vi "main.vi"() -> ()   [LabVIEW 2018]
uses:
  SubVIs_Dental robot/Type Define/Commmands.ctl
  SubVIs_Dental robot/Type Define/Main Pages.ctl
  <vilib>/Platform/TimedLoop/XDataNode/timing_clust.ctl
  <vilib>/Platform/TimedLoop/XDataNode/nitl_modes.ctl
  <vilib>/Platform/TimedLoop/XDataNode/wakeup.ctl
  <vilib>/Analysis/_algsub.llb/Vector Norm Type.ctl
  <vilib>/Analysis/baseanly.llb/A x Vector.vi
  a7223f14-2dee-44f5-bb18-0364424e4be1.vi
  0510b20e-cdd4-4c00-a2e4-b6458116f7e6.vi
  6765c77a-608f-47a9-82f1-7d78e4eb0e2c.vi
  9b5042e6-a8af-4737-a7d5-6a0044b5b849.vi
  4ad8b042-512e-4ff8-852c-0cd1c3cad4b9.vi
  86f0d0e6-1215-4d7f-931e-98a8c43bff1f.vi
  f29c3c44-4b71-459f-8cb8-0042c545ba9a.vi
  d7c4ca3e-ecce-44e0-a421-952e676fecf6.vi
  981894b4-ccec-4f9d-89cc-fdaa1394f8a6.vi
  9c9e3e7b-044e-4f20-b28a-2f2dc11135a4.vi
  9fd7527a-2d21-4efb-8458-bb367c16f289.vi
  ac7faa24-f845-40ca-90b7-81be7ed5a357.vi
  b63aa834-2712-49f4-8037-f59c6ffc9581.vi
  f501b187-2088-4d7b-8b35-1f4e4e40070a.vi
  <vilib>/Analysis/_algsub.llb/Real Vector Norm.vi
  bbe701d4-6856-4238-8169-f1a63681c652.vi
  2e5cd8ad-a022-48e3-a566-60a3cbf6d178.vi
  11c04ccb-2e07-4f2a-b784-9dc4474bd3c3.vi
  df89aa8a-d510-48a8-89d6-09f8ad9d1347.vi
  c9b8846e-2642-4342-81ce-7650c1843fd3.vi
  e93a78a8-cf73-409a-8246-49de62ed042d.vi
  3db6b772-aa7e-4faf-b327-bcfc711d862c.vi
  947c7df0-b853-4919-9a27-33aee5587755.vi
  376b9600-9bf4-49ac-95b6-11595f89b64b.vi
  2f109b7a-7238-4649-a91e-82c40714c455.vi
  015dea3f-de33-43d8-ac62-f4291712486d.vi
  365726ef-1bf1-41fb-8d10-812960490415.vi
  <vilib>/Platform/TimedLoop/XDataNode/loadnilvce.vi
  <vilib>/FPGAPlugInAG/PCIe-7841R/niLvFpga_Open_PCIe-7841R.vi
  <vilib>/rvi/interface/common/dynamic/niFpgaDynamicAddResources.vi
  <vilib>/Utility/error.llb/Error Cluster From Error Code.vi
  <vilib>/rvi/errors/niLvFpgaAdjustHostInterfaceError.vi
  Global Variables/Sensor_m.vi
  Global Variables/File_Torque.vi
  Global Variables/Fz_des.vi
  Global Variables/Sensor_Force.vi
  Global Variables/Command_Velocity.vi
  Global Variables/Command_Position.vi
  Global Variables/Sensor_Impluse.vi
  <vilib>/FPGAPlugInAG/Dynamic/niLvFpga_Close_Dynamic.vi
  <vilib>/Platform/TimedLoop/XDataNode/XDataNode.xnode
  <vilib>/rvi/interface/nirviOpenFPGA/nirviOpenFPGA.xnode
  FPGA Bitfiles/DentalRobotEther_FPGATarget_FPGA_dxM2ySpCtLw.lvbitx
  FPGA/FPGA.vi
  <vilib>/rvi/interface/nirviReadWriteControl/nirviReadWriteControl.xnode
  <vilib>/rvi/interface/nirviCloseFPGA/nirviCloseFPGA.xnode
  <vilib>/Platform/TimedLoop/XDataNode/XDNodeRunTimeDep.lvlib
  <vilib>/rvi/interface/Simulation/niFpgaSimulationCallBeginRW.vi
  <resource>/objmgr/IndComECAT.rc
  <vilib>/Analysis/NI_AALBase.lvlib
  <vilib>/Analysis/NI_AALPro.lvlib
  Global Variables/Demo_forces.vi
  4dd33180-7ea2-4f01-82c4-c6e235ae8763.vi
  9973e808-26c0-4418-8a5b-874f4b752693.vi
  1f0ace2b-62cd-4642-bc5f-9879a45fe932.vi
  8dd49e7d-a3e5-491e-87e0-138620dfdc3b.vi
  NiFpgaLv.dll
panel:
  out "A":dbl
  out "Torque (mNm)":dbl format="%#.2f"
  out "Rt_S":dbl[][](array[numeric])
  out "Start Points 2":T1 {"Z£c" format="%.3f"; "Y£c" format="%.3f"; "X£c" format="%.3f"; "Z" format="%.3f"; "Y" format="%.3f"; "X" format="%.3f"}
  out "scan engine":u32=10000
  out "External force_{t}":T2 {"£nez" format="%.3f"; "£ney" format="%.3f"; "£nex" format="%.3f"; "Fez" format="%.2f"; "Fey" format="%.2f"; "Fex" format="%.2f"}
  out "Finished_late":u32
  in  "Sensor Transform":bool
  out "DC mode":bool[](array[boolean])
  out "Slave State":u32(ring) items=["UNKNOWN"=0, "Init"=1, "PreOP"=2, "BootStrap"=3, "SafeOP"=4, "OP"=8]
  out "Error code":u16
  out "Control loop":u32
  out "Acceration":cluster{"X":i32, "Y":i32, "Z":i32}
  out "Torque Ratio":T3 {"Joint 6" format="%.3f"; "Joint 5" format="%.3f"; "Joint 4" format="%.3f"; "Joint 3" format="%.3f"; "Joint 2" format="%.3f"; "Joint 1" format="%.3f"}
  out "Joint Vel":T3 {"Joint 6" format="%.3f"; "Joint 5" format="%.3f"; "Joint 4" format="%.3f"; "Joint 3" format="%.3f"; "Joint 2" format="%.3f"; "Joint 1" format="%.3f"}
  out "Monitor loop":u32
  out "Position":T1 {"Z£c" format="%.3f"; "Y£c" format="%.3f"; "X£c" format="%.3f"; "Z" format="%.3f"; "Y" format="%.3f"; "X" format="%.3f"}
  out "Joints(degree)":T3 {"Joint 6" format="%.3f"; "Joint 5" format="%.3f"; "Joint 4" format="%.3f"; "Joint 3" format="%.3f"; "Joint 2" format="%.3f"; "Joint 1" format="%.3f"}
  out "Motion Status":T4
  out "Robot Status":T5
  out "Sensor_err":bool
  in  "Flags":enum16{"Intro", "Homing", "Autotune"}(ring)
  out "theta(degree)":dbl format="%.3f"
  out "Weight (g)":dbl format="%.3f"
  in  "Zeroing":bool
  out "External force_{S}":T2 {"£nez" format="%.3f"; "£ney" format="%.3f"; "£nex" format="%.3f"; "Fez" format="%.2f"; "Fey" format="%.2f"; "Fex" format="%.2f"}
  out "Sensor":T6 {"£nz" format="%.3f"; "£ny" format="%.3f"; "£nx" format="%.3f"; "Fz" format="%.2f"; "Fy" format="%.2f"; "Fx" format="%.2f"}
  out "V":dbl
  out "Instance":T7={"x"=0.01109137617807713, "y"=-0.0008918407815229689, "z"=0.01571725979663983, "£c"=-0.008503543554386012, " Fxo"=1.274069639052308, " Fyo"=-1.8630751344367247, " Fzo"=2.593164242802932, "Mxo"=-0.011336059591235648, "Myo"=-0.02215413804123321, "Mzo"=0.012300793701532243, "G"=1.5679867760034736} {"z" format="%.2f"; "G" format="%.3f"; "Mzo" format="%.3f"; "Myo" format="%.3f"; "Mxo" format="%.2f"; "Fzo" format="%.3f"; "Fyo" format="%.3f"; "Fxo" format="%.3f"; "£c" format="%.2f"; "y" format="%.2f"; "x" format="%.2f"}
  in  "Counter":i32
  out "Motions":dbl[][](array[numeric])
  out "Toqrues(plot)":dbl(graph)
  out "Forces(plot)":cluster{"Fex":dbl, "Fey":dbl, "Fez":dbl}(graph)
  out "Torques(plot)":cluster{" £nex":dbl, " £ney":dbl, " £nez":dbl}(graph)
  out "Finished_late":u32
  in  "Waiting":bool
  in  "Intro":bool
  out "Adm_joints":dbl[](array[numeric]) format="%.6f"
  in  "PID Gains":cluster{"Kp":dbl, "Kd":dbl, "Ki":dbl}={"Kp"=1.0, "Kd"=0.001, "Ki"=0.0}
  in  "threshold":sgl=3.0
  in  "Saturation":dbl[](array[numeric])=[-10.0, 10.0]
  in  "Kp":sgl
  in  "help":bool
  in  "Pause":bool
  in  "Reset":bool
  out "ERROR":string
  in  "Activate":bool
  in  "Home":bool
  in  "Set":bool
  in  "stop":bool
  in  "Setting":bool
  in  "RCT":bool
  in  "Dragging":bool
  in  "Jogging":bool
  in  "Pos Ctrl":bool
  in  "Joint Ctrl":bool
  in  "Pages":T8(tab)
  in  "Joints":sgl[](array[numeric])=[0.0, 0.0, 0.0, 0.0, 0.0, 0.0] step=1 format="%.3f"
  in  "Pos":sgl[](array[numeric]) step=1 format="%.3f"
  in  "Option":enum32{"Item 0", "Item 1"}(radio) caption="Radio Buttons"
  in  "Speed Ratio":i8=20 min=0 max=100 step=5
  in  "Jogging Ctrl":T9
  out "Moving?":bool
  out "Position":T1 {"Z£c" format="%.3f"; "Y£c" format="%.3f"; "X£c" format="%.3f"; "Z" format="%.3f"; "Y" format="%.3f"; "X" format="%.3f"}
  in  "Drag":bool
  in  "Autotune":bool
  in  "Mode":string(combo)="Custom"
  in  "TCP":enum32{"Long file", "Short file"}(tab)
  in  "Search_Long":bool
  in  "Long":T10
  out "Record":bool[](array[boolean])
  in  "Search_Rotation":bool
  in  "Short":T10
  out "Record":bool[](array[boolean])
  in  "Setting":bool
  in  "Step3":bool
  in  "Step2":bool
  in  "Step1":bool
  out "Demo subpages":T11(tab)
  in  "Done":bool
  in  "plan":bool
  in  "Root length":dbl=10.0 step=1000.0
  in  "Exp-Rep":bool
  in  "Compemsation":bool
  in  "Commands 2":u16(ring)=4 items=["MoveJoints"=1, "MovePose"=2, "MoveLin"=3, "MoveLinRelTRF"=4, "MoveLinRelWRF"=5, "Delay"=6, "SetBlending"=7, "SetJointVel"=8, "SetJointAcc"=9, "SetCartAngVel"=10, "SetCartLinVel"=11, "SetCartAcc"=12, "SetTRF"=13, "SetWRF"=14, "SetConf"=15, "SetAutoConf"=16, "SetCheckpoint"=17, "Gripper"=18, "SetGripperVel"=19, "SetGripperForce"=20, "MoveJointsVel"=21, "MoveLinVelWRF"=22, "MoveLinVelTRF"=23, "SetVelTimeout"=24]
  in  "Times":i32=5 step=1000
  in  "Seccction length":dbl=1.0 step=1000.0
  in  "limit_mA":dbl=75.0
  in  "Filter":u16(ring)=3 items=["Filter1", "Filter2", "Filter3", "Filter4"]
  in  "Calibration":u16(ring) items=["SI-20-1", "SI-40-2"]
  in  "Intro":bool
  in  "Sensor_tansform":i32[](array[numeric])=[0, 0, 0, 0, 0, 0] step=1
  in  "Setting_Joints":cluster{"SetJointVel":sgl, "SetJointAcc":sgl}={"SetJointVel"=60.0, "SetJointAcc"=150.0} {"SetJointAcc" min=0.001 max=150 step=5 format="%#.3f"; "SetJointVel" min=0.001 max=100 step=5 format="%#.3f"}
  in  "Setting_Others":T12={"SetBlending"=100.0, "SetAutoConf"=1.0, "SetVelTimeout"=0.002} {"SetVelTimeout" min=0.001 max=100 step=5 format="%#.3f"; "SetAutoConf" min=0 max=1 step=1; "SetBlending" min=0 max=100 step=5}
  in  "Setting_Cart":T13={"SetCartAngVel"=45.0, "SetCartLinVel"=3.0, "SetCartAcc"=600.0} {"SetCartAcc" min=0.001 max=600 step=5 format="%#.3f"; "SetCartLinVel" min=0.001 max=1000 step=5 format="%#_3f"; "SetCartAngVel" min=0.001 max=300 step=5 format="%#.3f"}
  in  "SetConf":sgl[](array[numeric])=[1.0, 1.0, 1.0] min=-1 max=1 step=2
  in  "SetWRF":sgl[](array[numeric])=[0.0, 0.0, 0.0, 0.0, 0.0, 0.0] step=1 format="%.3f"
  in  "Motion Control":T14
  in  "Sim Mode":bool
  in  "SetTRF":sgl[](array[numeric])=[79.370895, -0.46751443, 77.955, 1.2242525, -1.8750256, 0.0] step=1 format="%.3f"
  out "Showbar":bool
  out "Activating...":bool caption="Calibrating..."
  in  "Count avg":bool
  in  "T_avg":dbl=5.2
  in  "Pages":enum32{"Parameter Setting", "Tool Control"}(tab)
  in  "Pamameters setting":enum32{"Admittance Setting", "Tool Setting"}(tab)
  in  "Bi":dbl[](array[numeric])=[80.0, 80.0, 80.0, 160.0, 160.0, 160.0] step=0.1
  out "Mi":dbl[](array[numeric])=[0.0012, 0.0006, 0.0010999999999999998, 0.0017, 0.004, 0.0029000000000000002] step=0.0001
  in  "k":dbl=60.0 step=10000.0
  in  "Threshold":dbl[](array[numeric])=[0.1, 0.1, 0.1, 0.01, 0.01, 0.01] step=0.1
  in  "inverse(degree)":i32=270
  in  "PID":cluster{"Kp":dbl, "Kd":dbl, "Ki":dbl}={"Kp"=0.002, "Kd"=0.007, "Ki"=9e-05}
  in  "Count/revolution":i32=17408
  in  "Page_Motor":T15(tab)
  in  "PID_File feedrate":cluster{"Kp":dbl, "Kd":dbl, "Ki":dbl}={"Kp"=0.2, "Kd"=0.0, "Ki"=0.0}
  in  "Back_force":dbl=-2.0
  in  "Torque_des":dbl=30.0
  in  "Clear":bool
  out "Inverse Count":i32
  in  "Desired RPM":dbl=200.0 step=10.0 format="%.1f"
  out "Real RPM":dbl format="%.1f"
  in  "DIR4":bool=TRUE
  in  "Rotate":bool=TRUE
  in  "DC":fxp<+,32,0>=0.5
  in  "temp":i32
  in  "Inv":bool
  in  "wait":i32
  out "Torque (mNm) 2":dbl[](array[numeric]) format="%.1f"
  out "x*y":dbl[](array[numeric])
  out "Impulse(J)":dbl[](array[numeric])
  in  "Saturation":dbl[](array[numeric])=[-0.1, 0.6]
  in  "Add":bool
  out "w":dbl[](array[numeric])
  in  "Bi 3":dbl[](array[numeric])=[0.10000000000000003, 0.10000000000000003, 0.3, 0.07, 0.07, 0.15000000000000002] step=0.1
  in  "time constant":dbl=0.002 step=1000.0
  out "Sampling time (s)":dbl=0.002
  out "£c":dbl[](array[numeric])
  out "Vel_{t} (mm/s)":dbl[](array[numeric])
  out "Pos_{t} (mm)":dbl[](array[numeric])
  in  "F_des":dbl[](array[numeric])=[0.0, 0.0, 0.0, 0.0, 0.0, 0.0] step=0.1
  in  "Joints' Tor":bool
  out "Torques":T16(graph)
  out "store":fxp<+,32,0>[](array[numeric])
  # "ATI-mini40"
  # "Tool"
  # "Meca500"
  # "Finished_late"
  # "-175 ~ 175"
  # "Joint 1"
  # "Joint 2"
  # "-70 ~ 90"
  # "Joint 3"
  # "-135 ~ 70"
  # "Joint 4"
  # "-170 ~ 170"
  # "Joint 5"
  # "-170 ~ 170"
  # "Joint 6"
  # "-180 ~ 180"
  # "X"
  # "Y"
  # "Z"
  # "X£c"
  # "Y£c"
  # "Z£c"
  # "Max Velocity\nX, Y, Z           :    1000  mm/s\nX£c, Y£c, Z£c  :   300  deg/s"
  # "X"
  # "Y"
  # "Z"
  # "X£c"
  # "Y£c"
  # "Z£c"
  # "Sensor \nCompensation"
  # "long file"
  # "Short file"
  # "Tool Control"
  # "RCT procedure"
  # "Move to the injured tooth"
  # "Determine the length of the tooth root"
  # "Preoperative preparation is ready"
  # "Path Planning"
  # "Joints"
  # "Others"
  # "Cartesian"
  # "Motion Control"
  # "RCT procedure"
  # "Setting (Developer mode)"
  # "Tool Setting"
  # "OTR Setting"
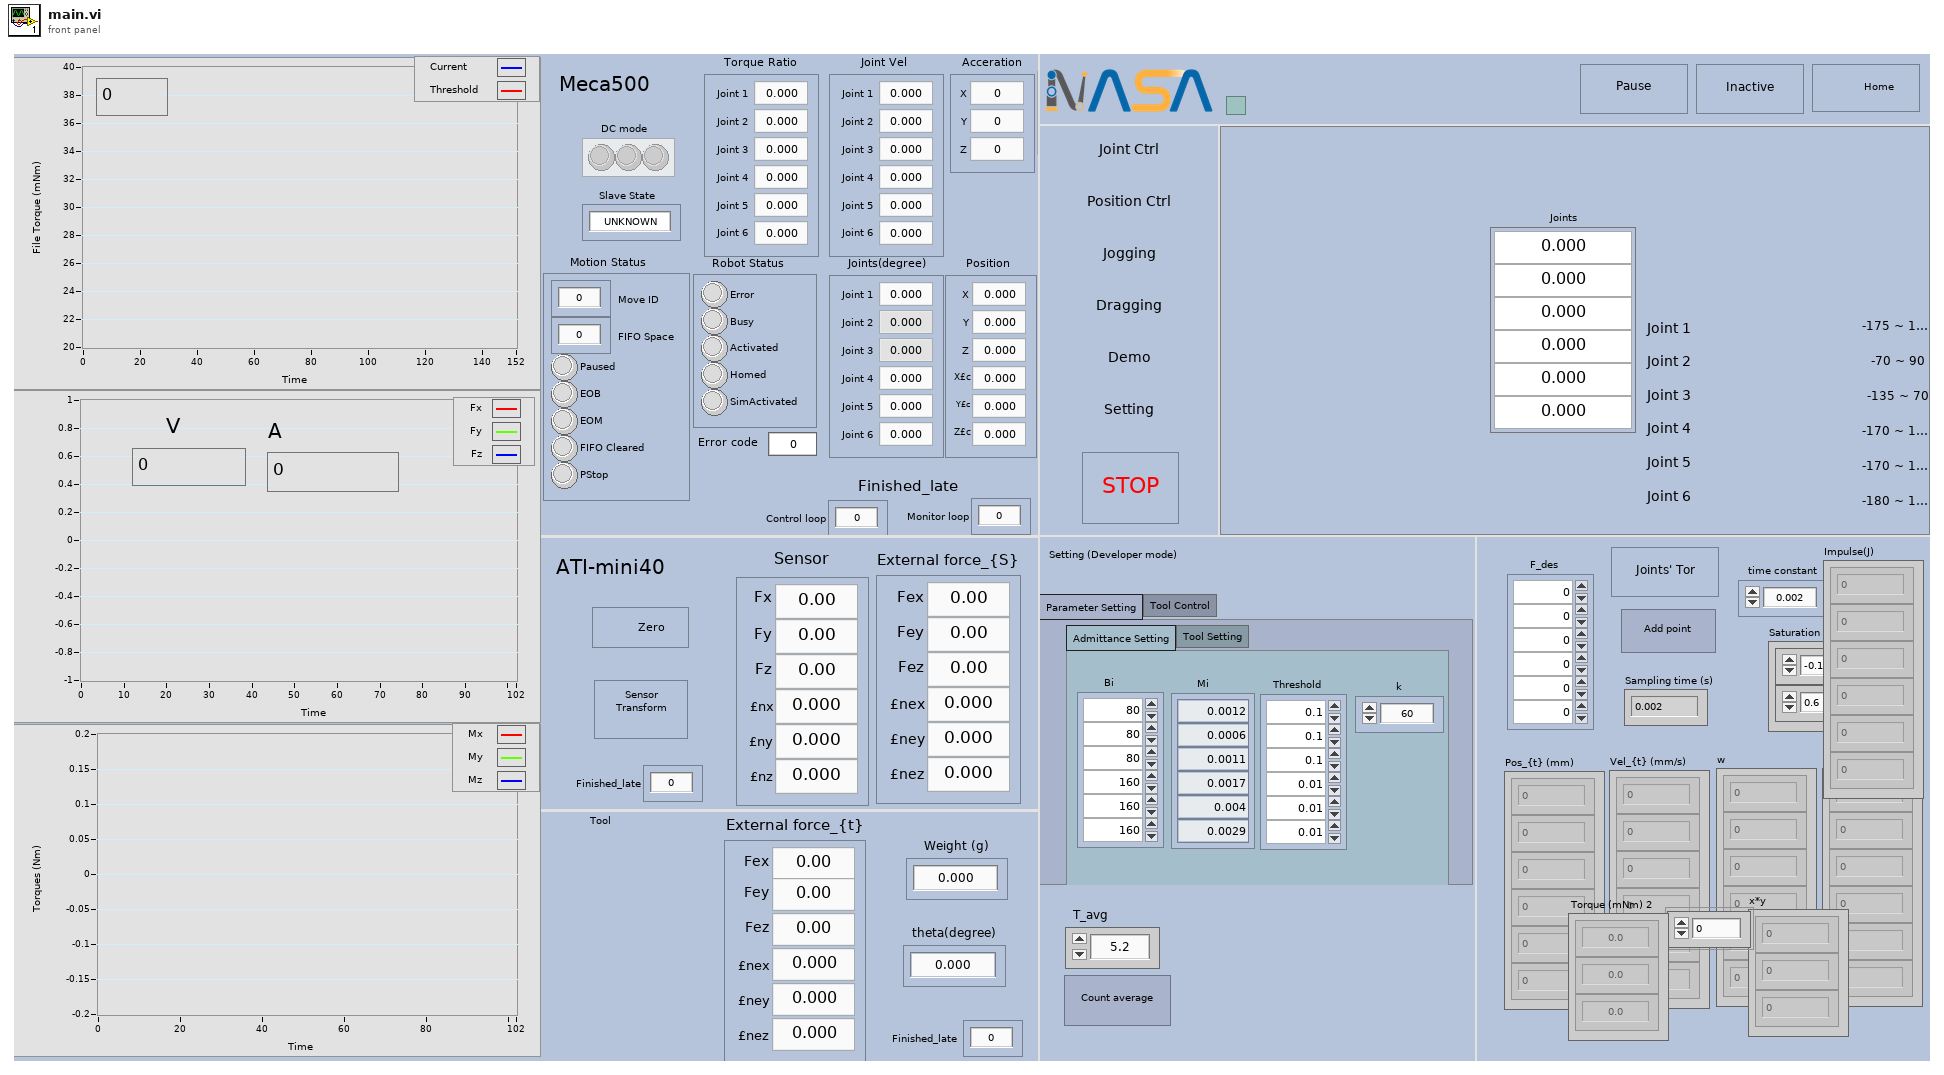
[diagram p1: front panel]
types:
  T1 = cluster{"X":sgl, "Y":sgl, "Z":sgl, "X£c":sgl, "Y£c":sgl, "Z£c":sgl}
  T2 = cluster{"Fex":dbl, "Fey":dbl, "Fez":dbl, " £nex":dbl, " £ney":dbl, " £nez":dbl}
  T3 = cluster{"Joint 1":sgl, "Joint 2":sgl, "Joint 3":sgl, "Joint 4":sgl, "Joint 5":sgl, "Joint 6":sgl}
  T4 = cluster{"Move ID":dbl, "FIFO Space":dbl, "Paused":bool, "EOB":bool, "EOM":bool, "FIFO Cleared":bool, "PStop":bool}
  T5 = cluster{"Error":bool, "Busy":bool, "Activated":bool, "Homed":bool, "SimActivated":bool}
  T6 = cluster{"Fx":dbl, "Fy":dbl, "Fz":dbl, " £nx":dbl, " £ny":dbl, " £nz":dbl}
  T7 = cluster{"x":dbl, "y":dbl, "z":dbl, "£c":dbl, " Fxo":dbl, " Fyo":dbl, " Fzo":dbl, "Mxo":dbl, "Myo":dbl, "Mzo":dbl, "G":dbl}
  T8 = enum32{"Joint", "Position", "Jogging", "Dragging", "Demo", "Setting", "Intro", "Waiting"}
  T9 = cluster{"Add Button":bool, "Add Button 2":bool, "Add Button 3":bool, "Add Button 4":bool, "Add Button 5":bool, "Add Button 6":bool, "Remove Button":bool, "Remove Button 2":bool, "Remove Button 3":bool, "Remove Button 4":bool, "Remove Button 5":bool, "Remove Button 6":bool}
  T10 = cluster{"Save Pos 1":bool, "Save Pos 2":bool, "Save Pos 3":bool, "Save Pos 4":bool}
  T11 = enum32{"Intro", "Step 1", "Step 2", "Step 3", "Setting"}
  T12 = cluster{"SetBlending":sgl, "SetAutoConf":sgl, "SetVelTimeout":sgl}
  T13 = cluster{"SetCartAngVel":sgl, "SetCartLinVel":sgl, "SetCartAcc":sgl}
  T14 = cluster{"Move ID":u16, "Clear Move":bool, "Reset PStop":bool}
  T15 = enum32{"Feedrate Ctrl", "OTR Ctrl", "Velocity Ctrl"}
  T16 = cluster{"Joint 1":sgl, "Joint2 ":sgl, "Joint 3":sgl, "Joint 4":sgl, "Joint 5":sgl, "Joint 6":sgl}
  T17 = typedef "Main Pages.ctl" = enum32{"Joint", "Position", "Jogging", "Dragging", "Demo", "Setting", "Intro", "Waiting"}
  T18 = typedef "Commmands.ctl" = enum16{"No command", "Movejoints", "MovePose", "MoveLin", "MoveLinRelTRF", "MoveLinRelWRF", "Delay", "SetBlending", "SetJointVel", "SetJointAcc", "SetCartAngVel", "SetCartLinVel", "SetCartAcc", "SetTRF", "SetWRF", "SetConf", "SetAutoConf", "SetCheckpoint", "Gripper", "SetGripperVel", "SetGripperForce", "MovejointsVel", "MoveLinVelWRF", "MoveLinVelTRF", "SetVelTimeout"}
  T19 = typedef "XDNodeRunTimeDep.lvlib/timing_clust.ctl" = cluster{"Expected End [f-1]":u64, "Actual End [f-1]":u64, "Finished Late? [f-1]":bool, "Expected End [i-1]":u64, "Actual End [i-1]":u64, "Finished Late? [i-1]":bool, "Expected Start [i]":u64, "Actual Start [i]":u64, "Expected Start [f]":u64, "Actual Start [f]":u64, "Source Name":string, "Structure Name":string, "Period":i64, "Deadline":i64, "Offset":i64, "Start":i64, "Priority":i32, "Timeout":i32, "Mode":T20, "Wakeup Reason":T21, "Error":errorcluster, "Source Type":string, "Secondary Source Type":string, "Global End Time":u64, "Global Start Time":u64, "Frame Duration":u64, "Iteration Duration":u64, "Assigned CPU":i32, "I/O Scan Engine Mode":u32}
  T20 = typedef "XDNodeRunTimeDep.lvlib/nitl_modes.ctl" = enum32{"No Change", "Process missed periods, maintain original phase", "Discard missed periods, maintain original phase", "Process missed periods, ignore original phase", "Discard missed periods, ignore original phase"}
  T21 = typedef "XDNodeRunTimeDep.lvlib/wakeup.ctl" = enum32{"Normal", "Aborted", "Asynchronous wakeup", "Timing source error", "Timed loop error", "Timeout"}
  T22 = enum32{"Without Ctrl", "OTR Ctrl", "Velocity Ctrl"}
  T23 = cluster{"Connector0/AI0":i16, "Connector0/AI1":i16, "Connector0/AI2":i16, "Connector0/AI3":i16, "Connector0/AI4":i16}
  T24 = typedef "NI_AALPro.lvlib/Vector Norm Type.ctl" = u16
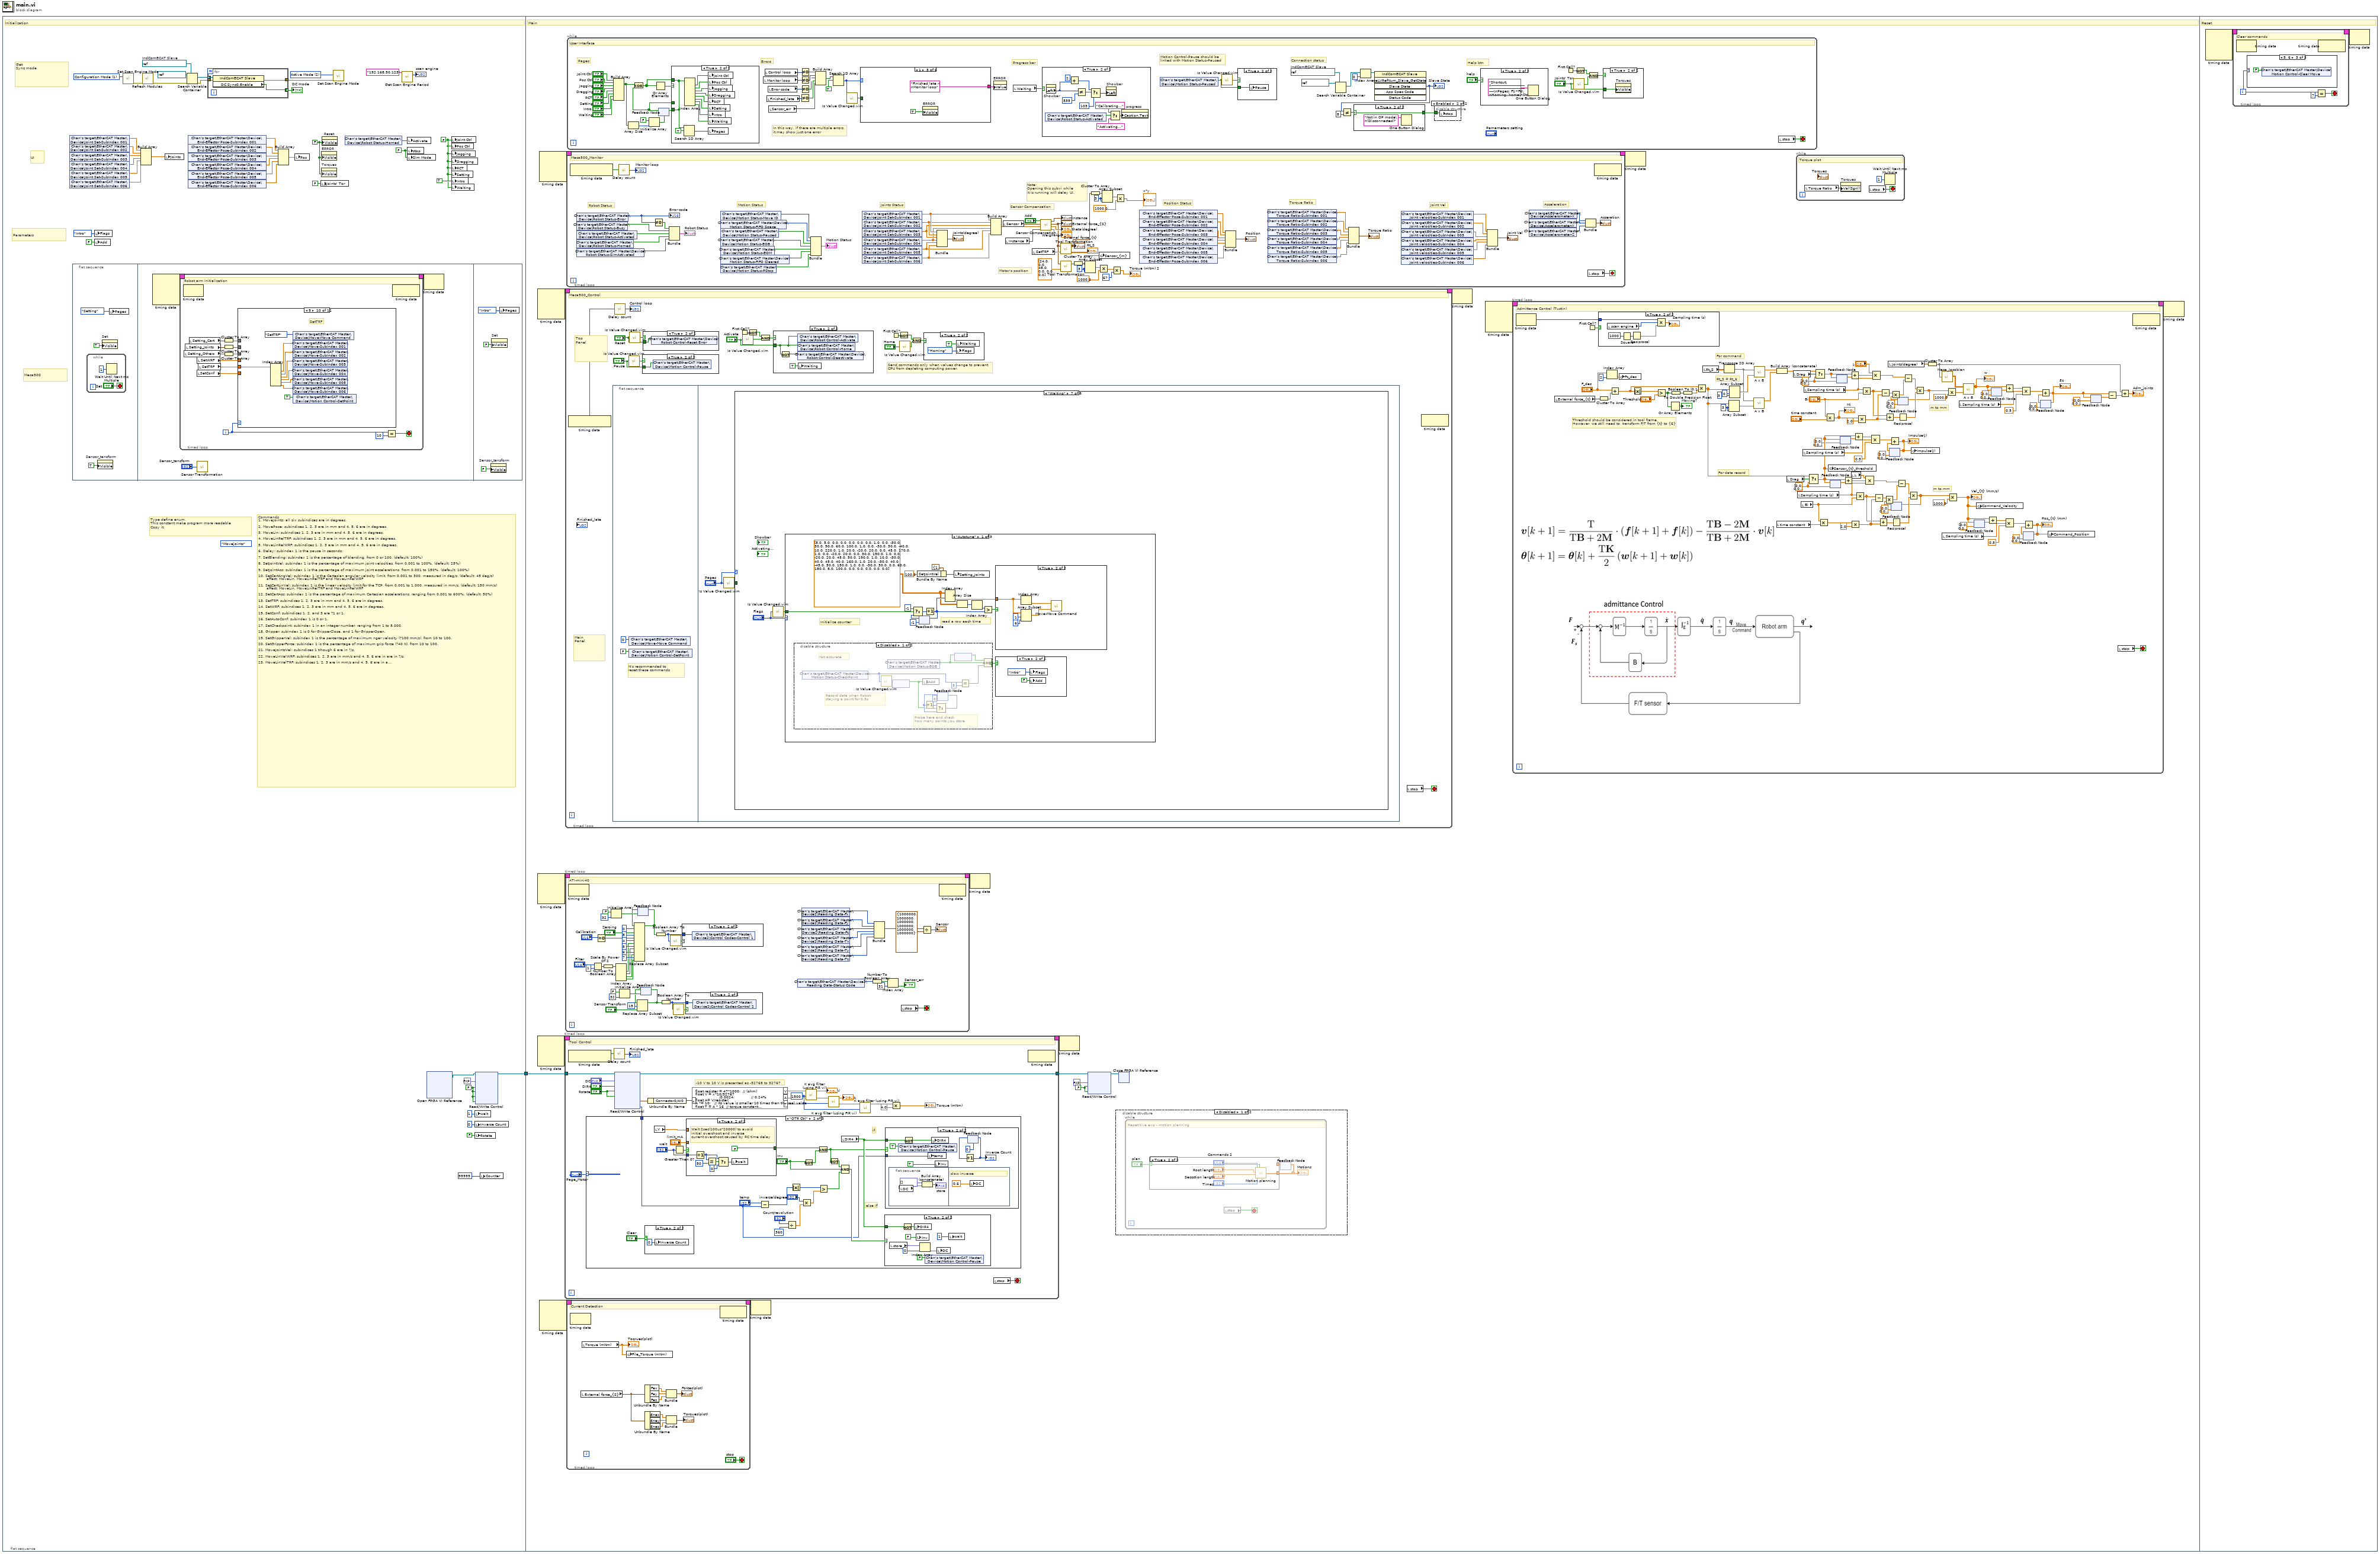
[diagram p0: block diagram]
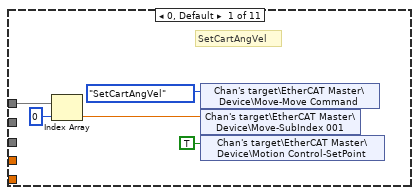
[diagram p2: hidden frame]
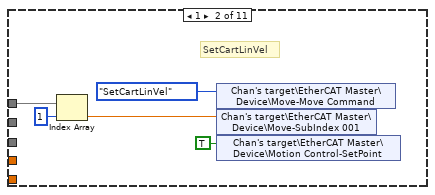
[diagram p3: hidden frame]
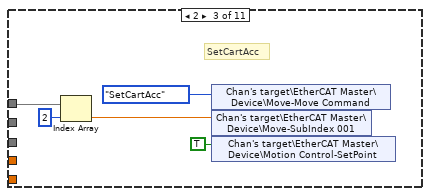
[diagram p4: hidden frame]
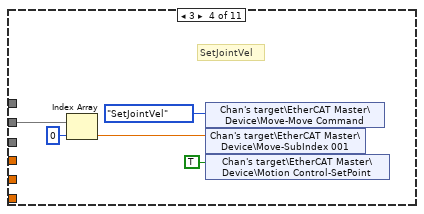
[diagram p5: hidden frame]
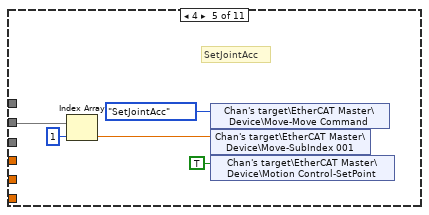
[diagram p6: hidden frame]
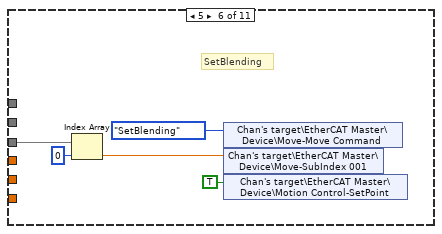
[diagram p7: hidden frame]
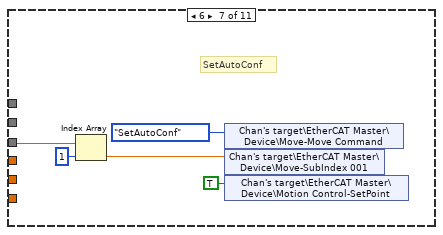
[diagram p8: hidden frame]
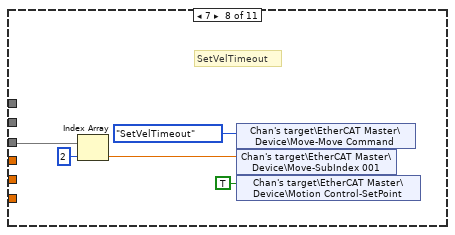
[diagram p9: hidden frame]
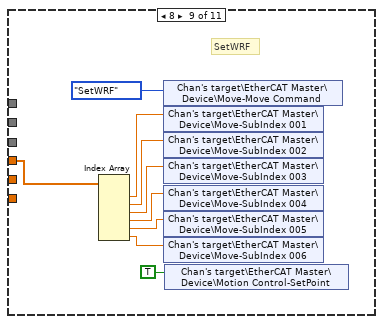
[diagram p10: hidden frame]
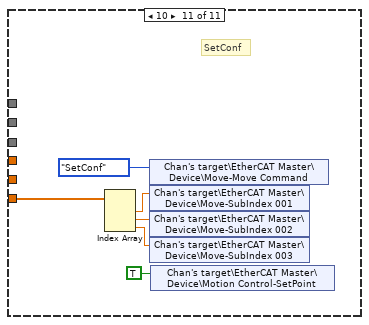
[diagram p11: hidden frame]
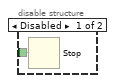
[diagram p18: hidden frame]
diagram:
  n1 = flat-sequence {
    tunnel: [w43] -> w1
    tunnel: w1 -> [w155]
    frame #0 {
      w11 = 2 items=["Configuration Mode"=1, "Active Mode"=2] ("mode (Active Mode)")
      w10 = 1 items=["Configuration Mode"=1, "Active Mode"=2] ("mode (Active Mode)")
      w9 = refnum<k21> refnum  # IndComECAT Slave
      (unwired) Commmands."Movejoints"
      w18 = FALSE ("stop")
      w35 = FALSE
      w6 = FALSE ("Visible")
      w41 = FALSE ("Reset4")
      # "Get\nSync mode"
      # "Meca500"
      # "Type define enum,\nThis constant make program more readable\nCopy it."
      # "Parameters"
      # "Commands\n1. MoveJoints: all six subindices are in degrees.\n\n2. MovePose: subindices 1, 2, 3 are in mm and 4, 5, 6 are in degrees.\n\n3. MoveLin: subindices 1, 2, 3 are in mm and 4, 5, 6 are in degrees.\n\n4. MoveLinRelTRF: subindices 1, 2, 3 are in mm and 4, 5, 6 are in degrees.\n\n5. MoveLinRelWRF: subindices 1, 2, 3 are in mm and 4, 5, 6 are in degrees.\n\n6. Delay: subindex 1 is the pause in seconds.\n\n7. SetBlending: subindex 1 is the percentage of blending, from 0 or 100. (default: 100%)\n\n8. SetJointVel: subindex 1 is the percentage of maximum joint velocities, from 0.001 to 100%. (default: 25%)\n\n9. SetJointAcc: subindex 1 is the percentage of maximum joint accelerations, from 0.001 to 150%. (default: 100%)\n\n10. SetCartAngVel: subindex 1 is the Cartesian angular velocity limit, from 0.001 to 300, measured in deg/s. (default: 45 deg/s)\n       affect: MoveLin, MoveLinRelTRF and MoveLinRelWRF\n\n11. SetCartLinVel: subindex 1 is the linear velocity limit for the TCP, from 0.001 to 1,000, measured in mm/s. (default: 150 mm/s)\n       affect: MoveLin, MoveLinRelTRF and MoveLinRelWRF\n\n12. SetCartAcc: subindex 1 is the percentage of maximum Cartesian accelerations, ranging from 0.001 to 600%. (default: 50%)\n\n13. SetTRF: subindices 1, 2, 3 are in mm and 4, 5, 6 are in degrees.\n\n14. SetWRF: subindices 1, 2, 3 are in mm and 4, 5, 6 are in degrees.\n\n15. SetConf: subindices 1, 2, and 3 are ?1 or 1.\n\n16. SetAutoConf: subindex 1 is 0 or 1.\n\n17. SetCheckpoint: subindex 1 in an integer number, ranging from 1 to 8,000.\n\n18. Gripper: subindex 1 is 0 for GripperClose, and 1 for GripperOpen.\n\n19. SetGripperVel: subindex 1 is the percentage of maximum nger velocity (?100 mm/s), from 10 to 100.\n\n20. SetGripperForce: subindex 1 is the percentage of maximum grip force (?40 N), from 10 to 100.\n\n21. MoveJointsVel: subindices 1 trhough 6 are in ?/s.\n\n22. MoveLinVelWRF: subindices 1, 2, 3 are in mm/s and 4, 5, 6 are in are in ?/s.\n\n23. MoveLinVelTRF: subindices 1, 2, 3 are in mm/s and 4, 5, 6 are in are in ?/s.\n\n24. SetVelTimeout: subindex 1 is in seconds, from 0.001 to 1s. (default: 0.050s)"
      # "UI"
      # "Initialization"
      n2 = shared-variable "Chan's target\\EtherCAT Master\\Device\\Joint Set-SubIndex 001"() -> (w28:sgl)  [unwired: 1 in, 1 out]
      n3 = shared-variable "Chan's target\\EtherCAT Master\\Device\\Joint Set-SubIndex 002"() -> (w33:sgl)  [unwired: 1 in, 1 out]
      n4 = shared-variable "Chan's target\\EtherCAT Master\\Device\\Joint Set-SubIndex 003"() -> (w32:sgl)  [unwired: 1 in, 1 out]
      n5 = shared-variable "Chan's target\\EtherCAT Master\\Device\\Joint Set-SubIndex 004"() -> (w31:sgl)  [unwired: 1 in, 1 out]
      n6 = shared-variable "Chan's target\\EtherCAT Master\\Device\\Joint Set-SubIndex 005"() -> (w30:sgl)  [unwired: 1 in, 1 out]
      n7 = shared-variable "Chan's target\\EtherCAT Master\\Device\\Joint Set-SubIndex 006"() -> (w29:sgl)  [unwired: 1 in, 1 out]
      n8 = flat-sequence {
        frame #0 {
          n9 = while {
            stop <- "Set" stop-if-true
            n10 = Wait Until Next ms Multiple(millisecond multiple=u32 1) -> ()  [unwired: 1 out]
          }
          n11 = property on="Sensor_tansform" class="Arr (strict)"("Visible"=TRUE) -> ()  [unwired: 2 in, 2 out]
          n12 = property on="Set" class="Bool"("Visible"=TRUE) -> ()  [unwired: 2 in, 2 out]
          n13 = local write "Pages"(Main_Pages."Setting" ("Pages")) -> ()
        }
        frame #1 {
          n14 = node-c288() -> (w55:T19)  [unwired: 4 in]
          n15 = timed-loop {
            timing: w55 -> [_]
            timing-out: [_] -> w54
            i -> [w66]
            stop <- w67 stop-if-true
            # "Robot arm initialization"
            n16 = node-c288() -> ()  [unwired: 1 in, 1 out]
            n17 = local read "Setting_Others"() -> (w62:T12)
            n18 = local read "Setting_Joints"() -> (w63:cluster{"SetJointVel":sgl, "SetJointAcc":sgl})
            n19 = local read "Setting_Cart"() -> (w65:T13)
            n20 = local read "SetConf"() -> (w57:sgl[])
            n21 = local read "SetWRF"() -> (w59:sgl[])
            n22 = local read "SetTRF"() -> (w58:sgl[])
            n23 = Cluster To Array(cluster=w65) -> (array=w64:sgl[])
            n24 = Cluster To Array(cluster=w63) -> (array=w60:sgl[])
            n25 = Cluster To Array(cluster=w62) -> (array=w61:sgl[])
            n26 = case shown="9" w66 {
              tunnel: w64 -> [w71 w75 w80 _ _ _ _ _ _ _ _]
              tunnel: w61 -> [_ _ _ _ _ w94 w99 w104 _ _ _]
              tunnel: w60 -> [_ _ _ w84 w89 _ _ _ _ _ _]
              tunnel: w59 -> [_ _ _ _ _ _ _ _ w109 _ _]
              tunnel: w58 -> [_ _ _ _ _ _ _ _ _ w118 _]
              tunnel: w57 -> [_ _ _ _ _ _ _ _ _ _ w127]
              frame 0, Default {
                # "SetCartAngVel"
                n27 = Index Array(array=w71, index=0) -> (element=w70:sgl)
                n28 = shared-variable "Chan's target\\EtherCAT Master\\Device\\Move-Move Command"(Commmands."SetCartAngVel") -> ()  [unwired: 1 in, 1 out]
                n29 = shared-variable "Chan's target\\EtherCAT Master\\Device\\Move-SubIndex 001"(w70) -> ()  [unwired: 1 in, 1 out]
                n30 = shared-variable "Chan's target\\EtherCAT Master\\Device\\Motion Control-SetPoint"(TRUE ("Motion Control-SetPoint")) -> ()  [unwired: 1 in, 1 out]
              }
              frame 1 {
                # "SetCartLinVel"
                n31 = Index Array(array=w75, index=1) -> (element=w76:sgl)
                n32 = shared-variable "Chan's target\\EtherCAT Master\\Device\\Move-Move Command"(Commmands."SetCartLinVel") -> ()  [unwired: 1 in, 1 out]
                n33 = shared-variable "Chan's target\\EtherCAT Master\\Device\\Move-SubIndex 001"(w76) -> ()  [unwired: 1 in, 1 out]
                n34 = shared-variable "Chan's target\\EtherCAT Master\\Device\\Motion Control-SetPoint"(TRUE ("Motion Control-SetPoint")) -> ()  [unwired: 1 in, 1 out]
              }
              frame 2 {
                # "SetCartAcc"
                n35 = Index Array(array=w80, index=2) -> (element=w81:sgl)
                n36 = shared-variable "Chan's target\\EtherCAT Master\\Device\\Move-Move Command"(Commmands."SetCartAcc") -> ()  [unwired: 1 in, 1 out]
                n37 = shared-variable "Chan's target\\EtherCAT Master\\Device\\Move-SubIndex 001"(w81) -> ()  [unwired: 1 in, 1 out]
                n38 = shared-variable "Chan's target\\EtherCAT Master\\Device\\Motion Control-SetPoint"(TRUE ("Motion Control-SetPoint")) -> ()  [unwired: 1 in, 1 out]
              }
              frame 3 {
                # "SetJointVel"
                n39 = Index Array(array=w84, index=0) -> (element=w86:sgl)
                n40 = shared-variable "Chan's target\\EtherCAT Master\\Device\\Move-Move Command"(Commmands."SetJointVel") -> ()  [unwired: 1 in, 1 out]
                n41 = shared-variable "Chan's target\\EtherCAT Master\\Device\\Move-SubIndex 001"(w86) -> ()  [unwired: 1 in, 1 out]
                n42 = shared-variable "Chan's target\\EtherCAT Master\\Device\\Motion Control-SetPoint"(TRUE ("Motion Control-SetPoint")) -> ()  [unwired: 1 in, 1 out]
              }
              frame 4 {
                # "SetJointAcc"
                n43 = Index Array(array=w89, index=1) -> (element=w91:sgl)
                n44 = shared-variable "Chan's target\\EtherCAT Master\\Device\\Move-Move Command"(Commmands."SetJointAcc") -> ()  [unwired: 1 in, 1 out]
                n45 = shared-variable "Chan's target\\EtherCAT Master\\Device\\Move-SubIndex 001"(w91) -> ()  [unwired: 1 in, 1 out]
                n46 = shared-variable "Chan's target\\EtherCAT Master\\Device\\Motion Control-SetPoint"(TRUE ("Motion Control-SetPoint")) -> ()  [unwired: 1 in, 1 out]
              }
              frame 5 {
                # "SetBlending"
                n47 = Index Array(array=w94, index=0) -> (element=w96:sgl)
                n48 = shared-variable "Chan's target\\EtherCAT Master\\Device\\Move-Move Command"(Commmands."SetBlending") -> ()  [unwired: 1 in, 1 out]
                n49 = shared-variable "Chan's target\\EtherCAT Master\\Device\\Move-SubIndex 001"(w96) -> ()  [unwired: 1 in, 1 out]
                n50 = shared-variable "Chan's target\\EtherCAT Master\\Device\\Motion Control-SetPoint"(TRUE ("Motion Control-SetPoint")) -> ()  [unwired: 1 in, 1 out]
              }
              frame 6 {
                # "SetAutoConf"
                n51 = Index Array(array=w99, index=1) -> (element=w101:sgl)
                n52 = shared-variable "Chan's target\\EtherCAT Master\\Device\\Move-Move Command"(Commmands."SetAutoConf") -> ()  [unwired: 1 in, 1 out]
                n53 = shared-variable "Chan's target\\EtherCAT Master\\Device\\Move-SubIndex 001"(w101) -> ()  [unwired: 1 in, 1 out]
                n54 = shared-variable "Chan's target\\EtherCAT Master\\Device\\Motion Control-SetPoint"(TRUE ("Motion Control-SetPoint")) -> ()  [unwired: 1 in, 1 out]
              }
              frame 7 {
                # "SetVelTimeout"
                n55 = Index Array(array=w104, index=2) -> (element=w106:sgl)
                n56 = shared-variable "Chan's target\\EtherCAT Master\\Device\\Move-Move Command"(Commmands."SetVelTimeout") -> ()  [unwired: 1 in, 1 out]
                n57 = shared-variable "Chan's target\\EtherCAT Master\\Device\\Move-SubIndex 001"(w106) -> ()  [unwired: 1 in, 1 out]
                n58 = shared-variable "Chan's target\\EtherCAT Master\\Device\\Motion Control-SetPoint"(TRUE ("Motion Control-SetPoint")) -> ()  [unwired: 1 in, 1 out]
              }
              frame 8 {
                # "SetWRF"
                n59 = Index Array(array=w109) -> (element #1=w116:sgl, element #2=w115:sgl, element #3=w114:sgl, element #4=w113:sgl, element #5=w112:sgl, element #6=w111:sgl)  [unwired: 6 in]
                n60 = shared-variable "Chan's target\\EtherCAT Master\\Device\\Move-Move Command"(Commmands."SetWRF") -> ()  [unwired: 1 in, 1 out]
                n61 = shared-variable "Chan's target\\EtherCAT Master\\Device\\Move-SubIndex 001"(w116) -> ()  [unwired: 1 in, 1 out]
                n62 = shared-variable "Chan's target\\EtherCAT Master\\Device\\Move-SubIndex 002"(w115) -> ()  [unwired: 1 in, 1 out]
                n63 = shared-variable "Chan's target\\EtherCAT Master\\Device\\Move-SubIndex 003"(w114) -> ()  [unwired: 1 in, 1 out]
                n64 = shared-variable "Chan's target\\EtherCAT Master\\Device\\Move-SubIndex 004"(w113) -> ()  [unwired: 1 in, 1 out]
                n65 = shared-variable "Chan's target\\EtherCAT Master\\Device\\Move-SubIndex 005"(w112) -> ()  [unwired: 1 in, 1 out]
                n66 = shared-variable "Chan's target\\EtherCAT Master\\Device\\Move-SubIndex 006"(w111) -> ()  [unwired: 1 in, 1 out]
                n67 = shared-variable "Chan's target\\EtherCAT Master\\Device\\Motion Control-SetPoint"(TRUE ("Motion Control-SetPoint")) -> ()  [unwired: 1 in, 1 out]
              }
              frame 9 {
                # "SetTRF"
                n68 = Index Array(array=w118) -> (element #1=w125:sgl, element #2=w124:sgl, element #3=w123:sgl, element #4=w122:sgl, element #5=w121:sgl, element #6=w120:sgl)  [unwired: 6 in]
                n69 = shared-variable "Chan's target\\EtherCAT Master\\Device\\Move-Move Command"(Commmands."SetTRF") -> ()  [unwired: 1 in, 1 out]
                n70 = shared-variable "Chan's target\\EtherCAT Master\\Device\\Move-SubIndex 001"(w125) -> ()  [unwired: 1 in, 1 out]
                n71 = shared-variable "Chan's target\\EtherCAT Master\\Device\\Move-SubIndex 002"(w124) -> ()  [unwired: 1 in, 1 out]
                n72 = shared-variable "Chan's target\\EtherCAT Master\\Device\\Move-SubIndex 003"(w123) -> ()  [unwired: 1 in, 1 out]
                n73 = shared-variable "Chan's target\\EtherCAT Master\\Device\\Move-SubIndex 004"(w122) -> ()  [unwired: 1 in, 1 out]
                n74 = shared-variable "Chan's target\\EtherCAT Master\\Device\\Move-SubIndex 005"(w121) -> ()  [unwired: 1 in, 1 out]
                n75 = shared-variable "Chan's target\\EtherCAT Master\\Device\\Move-SubIndex 006"(w120) -> ()  [unwired: 1 in, 1 out]
                n76 = shared-variable "Chan's target\\EtherCAT Master\\Device\\Motion Control-SetPoint"(TRUE ("Motion Control-SetPoint")) -> ()  [unwired: 1 in, 1 out]
              }
              frame 10 {
                # "SetConf"
                n77 = Index Array(array=w127) -> (element #1=w131:sgl, element #2=w130:sgl, element #3=w129:sgl)  [unwired: 3 in]
                n78 = shared-variable "Chan's target\\EtherCAT Master\\Device\\Move-Move Command"(Commmands."SetConf") -> ()  [unwired: 1 in, 1 out]
                n79 = shared-variable "Chan's target\\EtherCAT Master\\Device\\Move-SubIndex 001"(w131) -> ()  [unwired: 1 in, 1 out]
                n80 = shared-variable "Chan's target\\EtherCAT Master\\Device\\Move-SubIndex 002"(w130) -> ()  [unwired: 1 in, 1 out]
                n81 = shared-variable "Chan's target\\EtherCAT Master\\Device\\Move-SubIndex 003"(w129) -> ()  [unwired: 1 in, 1 out]
                n82 = shared-variable "Chan's target\\EtherCAT Master\\Device\\Motion Control-SetPoint"(TRUE ("Motion Control-SetPoint")) -> ()  [unwired: 1 in, 1 out]
              }
            }
            n83 = Equal?(x=w66, y=10) -> (x = y?=w67:bool)
            n84 = node-c288() -> ()  [unwired: 1 in, 1 out]
          }
          n85 = call "Sensor Transformation.vi"("Array"="Sensor_tansform") -> ()
          n86 = node-c288(w54) -> ()  [unwired: 1 out]
        }
        frame #2 {
          n87 = property on="Sensor_tansform" class="Arr (strict)"("Visible"=FALSE) -> ()  [unwired: 2 in, 2 out]
          n88 = property on="Set" class="Bool"("Visible"=FALSE) -> ()  [unwired: 2 in, 2 out]
          n89 = local write "Pages"(Main_Pages."Intro" ("Pages")) -> ()
        }
      }
      n90 = local write "Flags"(enum16{"Intro", "Homing", "Autotune"}."Intro" ("Flags")) -> ()
      n91 = local write "Add"(FALSE ("Add")) -> ()
      n92 = call <vilib>:"Set Scan Engine Mode.vi"("mode (Active Mode)"=w10) -> ("error out"=w16:errorcluster)  [unwired: 14 in]
      n93 = Build Array(w28, w33, w32, w31, w30, w29) -> (w27:sgl[])
      n94 = call <vilib>:"Refresh Modules.vi"("error in (no error)"=w16) -> ("error out"=w17:errorcluster)  [unwired: 10 in]
      n95 = local write "Joints"(w27) -> ()
      n96 = Search Variable Container(7:w9, 8:w17, 11:refnum<k21> "ni.var.io:/" ("container refnum in")) -> (0:w14:errorcluster, 2:w15:refnum<k21>[])  [unwired: 3 in, 1 out]
      n97 = shared-variable "Chan's target\\EtherCAT Master\\Device\\End-Effector Pose-SubIndex 001"() -> (w26:sgl)  [unwired: 1 in, 1 out]
      n98 = shared-variable "Chan's target\\EtherCAT Master\\Device\\End-Effector Pose-SubIndex 002"() -> (w25:sgl)  [unwired: 1 in, 1 out]
      n99 = shared-variable "Chan's target\\EtherCAT Master\\Device\\End-Effector Pose-SubIndex 003"() -> (w24:sgl)  [unwired: 1 in, 1 out]
      n100 = shared-variable "Chan's target\\EtherCAT Master\\Device\\End-Effector Pose-SubIndex 004"() -> (w23:sgl)  [unwired: 1 in, 1 out]
      n101 = shared-variable "Chan's target\\EtherCAT Master\\Device\\End-Effector Pose-SubIndex 005"() -> (w22:sgl)  [unwired: 1 in, 1 out]
      n102 = shared-variable "Chan's target\\EtherCAT Master\\Device\\End-Effector Pose-SubIndex 006"() -> (w21:sgl)  [unwired: 1 in, 1 out]
      n103 = for {
        tunnel: w15 -> [w47] mode=indexing
        tunnel: w14 -> [w46]
        tunnel: [w45] -> w13
        tunnel: [w44] -> w12 mode=indexing
        n104 = property class="IndComECAT Slave"(reference=w47, error in=w46) -> (error out=w45:errorcluster, "DC.Sync0.Enable"=w44:bool)  [unwired: 1 out]
      }
      "DC mode" <- w12
      n105 = Build Array(w26, w25, w24, w23, w22, w21) -> (w20:sgl[])
      n106 = local write "Pos"(w20) -> ()
      n107 = local write "Joints' Tor"(FALSE ("Joints' Tor")) -> ()
      n108 = property on="ERROR" class="Str"("Visible"=w6) -> ()  [unwired: 2 in, 2 out]
      n109 = property on="Torques" class="WFChart (strict)"("Visible"=w6) -> ()  [unwired: 2 in, 2 out]
      n110 = property on="Reset" class="Bool"("Visible"=w6) -> ()  [unwired: 2 in, 2 out]
      n111 = call <vilib>:"Set Scan Engine Mode.vi"("mode (Active Mode)"=w11, "error in (no error)"=w13) -> ()  [unwired: 13 in, 1 out]
      n112 = shared-variable "Chan's target\\EtherCAT Master\\Device\\Robot Status-Homed"() -> (w37:bool)  [unwired: 1 in, 1 out]
      n113 = call <vilib>:"Get Scan Engine Period.vi"("target address (localhost)"="192.168.50.123") -> ("scan period (uSec)"=→"scan engine":u32)  [unwired: 13 in, 1 out]
      n114 = local write "Activate"(w37) -> ()
      n115 = local write "stop"(w18) -> ()
      n116 = local write "Sim Mode"(w18) -> ()
      n117 = xnode "Open FPGA VI Reference"() -> ("FPGA VI Reference Out"=w2:refnum<k20>)  [unwired: 2 in, 1 out]
      n118 = local write "Joint Ctrl"(w35) -> ()
      n119 = local write "Pos Ctrl"(w35) -> ()
      n120 = local write "Jogging"(w35) -> ()
      n121 = local write "Dragging"(w35) -> ()
      n122 = local write "RCT"(w35) -> ()
      n123 = local write "Setting"(w35) -> ()
      n124 = local write "Intro"(TRUE) -> ()
      n125 = local write "Waiting"(w35) -> ()
      n126 = local write "wait"(1 ("wait")) -> ()
      n127 = local write "Inverse Count"(0 ("Inverse Count")) -> ()
      n128 = local write "Rotate"(FALSE ("Rotate")) -> ()
      n129 = xnode "Read/Write Control"("FPGA VI Reference In"=w2, "CH2 DC"=fxp<+,32,0> 0.0 ("CH4 DC"), "Reset 1"=w41, "ENA1"=w41, "STBY1"=w41, "DIR1"=w41) -> ("FPGA VI Reference Out"=w43:refnum<k20>)  [unwired: 1 in, 1 out]
      n130 = local write "Counter"(99999 ("flag")) -> ()
    }
    frame #1 {
      w146 = FALSE ("ENA4")
      # "Main"
      n131 = node-c288() -> (w150:T19)  [unwired: 4 in]
      n132 = node-c288() -> (w154:T19)  [unwired: 4 in]
      n133 = node-c288() -> (w142:T19)  [unwired: 4 in]
      n134 = node-c288() -> (w152:T19)  [unwired: 4 in]
      n135 = node-c288() -> (w148:T19)  [unwired: 4 in]
      n136 = timed-loop {
        timing: w150 -> [_]
        timing-out: [_] -> w149
        tunnel: w155 -> [w486]
        tunnel: [w481] -> w144
        stop <- w479 stop-if-true
        w470 = 1500 ("avg num")
        # "-10 V to 10 V is presented as -32768 to 32767"
        # "Tool Control"
        n137 = node-c288() -> (w476:bool)  [unwired: 1 in]
        n138 = call "Delay count.vi"("Finished Late? [i-1]"=w476) -> ("Count"=→"Finished_late":u32)
        n139 = xnode "Read/Write Control"("FPGA VI Reference In"=w486, "CH1 DC"="DC", "DIR1"="DIR4", "STBY1"="Rotate", "ENA1"="Rotate") -> ("FPGA VI Reference Out"=w481:refnum<k20>, "Analog"=w483:T23, "Position 1"=w478:i32)  [unwired: 1 in, 1 out]
        n140 = case shown="\"OTR Ctrl\"" "Page_Motor" {
          tunnel: w478 -> [_ w489 w540]
          frame "Feedrate Ctrl", Default {
          }
          frame "OTR Ctrl" {
            # "else if"
            # "if"
            n141 = case shown="True" "Clear" {
              frame False {
              }
              frame True {
                n142 = local write "Inverse Count"(0 ("Inverse Count")) -> ()
              }
            }
            n143 = local read "V"() -> (w488:dbl)
            n144 = Greater Than 0?(x="wait") -> (x > 0?=w487:bool)
            n145 = case shown="True" w487 {
              tunnel: [w510 FALSE] -> w497
              tunnel: w488 -> [w512 _]
              tunnel: "limit_mA" -> [w511 _]
              tunnel: "wait" -> [_ w513]
              frame False {
                n146 = Greater?(x=w512, y=w511) -> (0:w510:bool)
              }
              frame True {
                # "Wait 2sec(100us*20000) to avoid \ninitial overshoot and inverse \ncurrent overshoot caused by RC time delay"
                n147 = Increment(x=w513) -> (x+1=w516:i32)
                n148 = Less Or Equal?(x=w516, y=50) -> (x <= y?=w515:bool)
                n149 = Select(t=w516, s=w515, f=0) -> (s? t:f=w517:i32)
                n150 = local write "wait"(w517) -> ()
              }
            }
            n151 = Subtract(x="temp", y=w489) -> (x-y=w506:i32)
            n152 = Divide(x="Count/revolution", y=360) -> (x/y=w499:dbl)
            n153 = Absolute Value(x=w506) -> (abs(x)=w496:i32)
            n154 = Multiply(x="inverse(degree)", y=w499) -> (x*y=w503:dbl)
            n155 = Not(x="Inv") -> (.not. x?=w508:bool)
            n156 = Greater?(x=w496, y=w503) -> (0:w494:bool)
            n157 = Compound Arithmetic op=AND(w497, w508) -> (w498:bool)
            n158 = Not(x=w498) -> (.not. x?=w507:bool)
            n159 = local read "DIR4"() -> (w502:bool)
            n160 = Compound Arithmetic op=AND(w507, "Inv", w494) -> (w492:bool)
            n161 = case shown="True" w492 {
              tunnel: w502 -> [_ w527]
              frame False {
              }
              frame True {
                n162 = local read "store"() -> (w522:fxp<+,32,0>[])
                n163 = Not(x=w527) -> (.not. x?=w526:bool)
                n164 = local write "DIR4"(w526) -> ()
                n165 = local write "Inv"(FALSE ("Inv")) -> ()
                n166 = Index Array(array=w522, index=0) -> (element=w523:fxp<+,32,0>)
                n167 = shared-variable "Chan's target\\EtherCAT Master\\Device\\Motion Control-Pause"(FALSE ("Motion Control-Pause")) -> ()  [unwired: 1 in, 1 out]
                n168 = local write "DC"(w523) -> ()
                n169 = local write "wait"(1 ("wait")) -> ()
              }
            }
            n170 = case shown="True" w498 {
              tunnel: w502 -> [_ w535]
              tunnel: w489 -> [_ w534]
              frame False {
              }
              frame True {
                n171 = flat-sequence {
                  frame #0 {
                    n172 = local read "DC"() -> (w536:fxp<+,32,0>)
                    n173 = Build Array (concatenate)(fxp<+,1,1>[] [], w536) -> (→"store":fxp<+,32,0>[])
                  }
                  frame #1 {
                    # "slow inverse"
                    n174 = local write "DC"(0.6) -> ()
                  }
                }
                n175 = shared-variable "Chan's target\\EtherCAT Master\\Device\\Motion Control-Pause"(TRUE ("Motion Control-Pause")) -> ()  [unwired: 1 in, 1 out]
                n176 = Not(x=w535) -> (.not. x?=w533:bool)
                n177 = local write "temp"(w534) -> ()
                n178 = local write "DIR4"(w533) -> ()
                n179 = local write "Inv"(TRUE ("Inv")) -> ()
                n180 = feedback #1(0) -> (w530:i32)
                n181 = Increment(x=w530) -> (x+1=w529:i32)
                "Inverse Count" <- w529
                n182 = feedback-in #1(w529) -> ()
              }
            }
          }
          frame "Velocity Ctrl" {
            n183 = feedback #2(0.0) -> (w545:dbl)
            n184 = call "PID r-y windup_chan.vi"("PID Gains"="PID", "Saturation"=dbl[] [-1.0, 1.0], "Reverse Motor?"=TRUE, "Encoder position"=w545, "Reference"="Desired RPM") -> ("DIR"=w543:bool, "Duty Cycle (Abs)"=w542:dbl)  [unwired: 3 in, 2 out]
            n185 = local write "DC"(w542) -> ()
            n186 = local write "DIR4"(w543) -> ()
            n187 = local read "Count/revolution"() -> (w556:i32)
            n188 = feedback #3(0 ("Position4")) -> (w549:i32)
            n189 = feedback-in #3(w540) -> ()
            n190 = Subtract(x=w549, y=w540) -> (x-y=w553:i32)
            n191 = Absolute Value(x=w553) -> (abs(x)=w552:i32)
            n192 = Sign(1:w553) -> (0:w554:i32)
            n193 = Divide(x=w552, y=w556) -> (x/y=w548:dbl)
            n194 = Compound Arithmetic op=MULTIPLY(120000.0 ("x"), w554, w548) -> (w557:dbl)
            "Real RPM" <- w557
            n195 = feedback-in #2(w557) -> ()
          }
        }
        n196 = Unbundle By Name(w483) -> ("Connector0/AI0"=w477:i16)
        n197 = formula code="float resister = 47*1000;  // (ohm)\nfloat V = x*10/32767                        \n                    /0.0024;              // 0.24%\nfloat A= V/resister;\nA *= 10;   // Its value is smaller 10 times than the real value\nfloat T = A * 16  // torque constant \n                     * 67; //  gear ratio"("x"=w477) -> ("A"=w472:dbl, "V"=w474:dbl, "T"=w469:dbl)
        n198 = call "K avg filter (using FIR vi).vi"("avg num"=w470, "x"=w474) -> ("Filtered x"=→"V":dbl)  [unwired: 9 in]
        n199 = call "K avg filter (using FIR vi).vi"("avg num"=w470, "x"=w472) -> ("Filtered x"=→"A":dbl)  [unwired: 9 in]
        n200 = call "K avg filter (using FIR vi).vi"("avg num"=w470, "x"=w469) -> ("Filtered x"=w468:dbl)  [unwired: 9 in]
        n201 = Multiply(x=w468, y=4.0) -> (x*y=→"Torque (mNm)":dbl)
        n202 = local read "stop"() -> (w479:bool)
        n203 = node-c288() -> ()  [unwired: 1 in, 1 out]
      }
      n204 = timed-loop {
        timing: w154 -> [_]
        timing-out: [_] -> w153
        stop <- w659 stop-if-true
        # "Main\nPanel"
        # "Send commands only when values change to prevent \nCPU from depleting computing power."
        # "Top\nPanel"
        # "Meca500_Control"
        n205 = node-c288() -> (w658:bool)  [unwired: 1 in]
        n206 = flat-sequence {
          frame #0 {
            # "It's recommended to \nreset these commands"
            n207 = shared-variable "Chan's target\\EtherCAT Master\\Device\\Move-Move Command"(u32 0 ("Move-Move Command")) -> ()  [unwired: 1 in, 1 out]
            n208 = shared-variable "Chan's target\\EtherCAT Master\\Device\\Motion Control-SetPoint"(FALSE ("Motion Control-SetPoint")) -> ()  [unwired: 1 in, 1 out]
          }
          frame #1 {
            n209 = call "Is Value Changed.vim"("value"="Pages") -> ("changed or first call?"=w663:bool)
            n210 = case shown="\"Waiting\"" "Pages" {
              tunnel: w663 -> [w664 w677 _ w733 w834 _ _ _]
              frame "Joint" {
                n211 = flat-sequence {
                  tunnel: w664 -> [w665]
                  frame #0 {
                    n212 = case shown="True" w665 {
                      frame False {
                      }
                      frame True {
                        # "Update the value when switching to this page."
                        n213 = shared-variable "Chan's target\\EtherCAT Master\\Device\\Joint Set-SubIndex 001"() -> (w666:sgl)  [unwired: 1 in, 1 out]
                        n214 = shared-variable "Chan's target\\EtherCAT Master\\Device\\Joint Set-SubIndex 002"() -> (w672:sgl)  [unwired: 1 in, 1 out]
                        n215 = shared-variable "Chan's target\\EtherCAT Master\\Device\\Joint Set-SubIndex 003"() -> (w671:sgl)  [unwired: 1 in, 1 out]
                        n216 = shared-variable "Chan's target\\EtherCAT Master\\Device\\Joint Set-SubIndex 004"() -> (w670:sgl)  [unwired: 1 in, 1 out]
                        n217 = shared-variable "Chan's target\\EtherCAT Master\\Device\\Joint Set-SubIndex 005"() -> (w669:sgl)  [unwired: 1 in, 1 out]
                        n218 = shared-variable "Chan's target\\EtherCAT Master\\Device\\Joint Set-SubIndex 006"() -> (w668:sgl)  [unwired: 1 in, 1 out]
                        n219 = Build Array(w666, w672, w671, w670, w669, w668) -> (w667:sgl[])
                        n220 = local write "Joints"(w667) -> ()
                      }
                    }
                  }
                  frame #1 {
                    n221 = call "Is Value Changed.vim"("value"="Joints") -> ("changed or first call?"=w673:bool)
                    n222 = case shown="True" w673 {
                      tunnel: "Joints" -> [_ w675]
                      frame False {
                      }
                      frame True {
                        n223 = call "Move-Move Command.vi"("Move-SubIndex"=w675, "Move-Move Command"=Commmands."Movejoints" ("Enum")) -> ()  [unwired: 1 in]
                      }
                    }
                  }
                }
              }
              frame "Position" {
                n224 = flat-sequence {
                  tunnel: w677 -> [w678]
                  frame #0 {
                    n225 = case shown="True" w678 {
                      frame False {
                      }
                      frame True {
                        # "Update the value when switching to this page."
                        n226 = shared-variable "Chan's target\\EtherCAT Master\\Device\\End-Effector Pose-SubIndex 001"() -> (w685:sgl)  [unwired: 1 in, 1 out]
                        n227 = shared-variable "Chan's target\\EtherCAT Master\\Device\\End-Effector Pose-SubIndex 002"() -> (w684:sgl)  [unwired: 1 in, 1 out]
                        n228 = shared-variable "Chan's target\\EtherCAT Master\\Device\\End-Effector Pose-SubIndex 003"() -> (w683:sgl)  [unwired: 1 in, 1 out]
                        n229 = shared-variable "Chan's target\\EtherCAT Master\\Device\\End-Effector Pose-SubIndex 004"() -> (w682:sgl)  [unwired: 1 in, 1 out]
                        n230 = shared-variable "Chan's target\\EtherCAT Master\\Device\\End-Effector Pose-SubIndex 005"() -> (w681:sgl)  [unwired: 1 in, 1 out]
                        n231 = shared-variable "Chan's target\\EtherCAT Master\\Device\\End-Effector Pose-SubIndex 006"() -> (w680:sgl)  [unwired: 1 in, 1 out]
                        n232 = Build Array(w685, w684, w683, w682, w681, w680) -> (w679:sgl[])
                        n233 = local write "Pos"(w679) -> ()
                      }
                    }
                  }
                  frame #1 {
                    n234 = call "Is Value Changed.vim"("value"="Pos") -> ("changed or first call?"=w686:bool)
                    n235 = case shown="True" w686 {
                      tunnel: "Pos" -> [_ w688]
                      frame False {
                      }
                      frame True {
                        n236 = call "Move-Move Command.vi"("Move-SubIndex"=w688, "Move-Move Command"=Commmands."MovePose" ("Enum")) -> ()  [unwired: 1 in]
                      }
                    }
                  }
                }
              }
              frame "Jogging" {
                # "Note:\n       Jogging is implemented by sending velocity command.\n       However, the Real Time module cannot use released mechanical action,     \n       so you can only click a button step by step instead of pressing it continuoesly."
                # "Watch out the order\nof this cluster"
                # "Max Vel\nX, Y, Z                  : 1000  mm/s\nX_£c, Y_£c, Z_£c  :   300  deg/s"
                n237 = Cluster To Array(cluster="Jogging Ctrl") -> (array=w694:bool[])
                n238 = Search 1D Array(1D array=w694, element=TRUE) -> (index of element=w710:i32)  [unwired: 1 in]
                n239 = Quotient & Remainder(x=w710, y=6) -> (x-y*floor(x/y)=w708:i32, floor(x/y)=w702:i32)
                n240 = To Double Precision Float(number="Speed Ratio") -> (double precision float=w711:dbl)
                n241 = Equal To 0?(x=w702) -> (x = 0?=w699:bool)
                n242 = Less?(x=w708, y=3) -> (x < y?=w706:bool)
                n243 = Select(t=1.0, s=w699, f=-1.0) -> (s? t:f=w698:dbl)
                n244 = Multiply(x=w711, y=0.01) -> (x*y=w701:dbl)
                n245 = Select(t=1000.0, s=w706, f=300.0) -> (s? t:f=w705:dbl)
                n246 = Compound Arithmetic op=MULTIPLY(w705, w698, w701) -> (w704:dbl)
                n247 = case shown="\"Item 0\", Default" "Option" {
                  tunnel: [Commmands."MoveLinVelWRF" ("Enum") Commmands."MoveLinVelTRF" ("Enum")] -> w717
                  frame "Item 0", Default {
                  }
                  frame "Item 1" {
                  }
                }
                n248 = Initialize Array(sgl 0.0, 6 ("dimension size")) -> (w690:sgl[])
                n249 = To Single Precision Float(number=w704) -> (single precision float=w712:sgl)
                n250 = Replace Array Subset(array=w690, new element=w712, index=w708) -> (w715:sgl[])
                n251 = Index Array(array=w715) -> (element #1=w719:sgl, element #2=w720:sgl, element #3=w721:sgl, element #4=w722:sgl, element #5=w723:sgl, element #6=w724:sgl)  [unwired: 6 in]
                n252 = Or Array Elements(Boolean array=w694) -> (logical OR=w718:bool)
                n253 = shared-variable "Chan's target\\EtherCAT Master\\Device\\Move-Move Command"(w717) -> ()  [unwired: 1 in, 1 out]
                n254 = shared-variable "Chan's target\\EtherCAT Master\\Device\\Move-SubIndex 001"(w719) -> ()  [unwired: 1 in, 1 out]
                n255 = shared-variable "Chan's target\\EtherCAT Master\\Device\\Move-SubIndex 002"(w720) -> ()  [unwired: 1 in, 1 out]
                n256 = shared-variable "Chan's target\\EtherCAT Master\\Device\\Move-SubIndex 003"(w721) -> ()  [unwired: 1 in, 1 out]
                n257 = shared-variable "Chan's target\\EtherCAT Master\\Device\\Move-SubIndex 004"(w722) -> ()  [unwired: 1 in, 1 out]
                n258 = shared-variable "Chan's target\\EtherCAT Master\\Device\\Move-SubIndex 005"(w723) -> ()  [unwired: 1 in, 1 out]
                n259 = shared-variable "Chan's target\\EtherCAT Master\\Device\\Move-SubIndex 006"(w724) -> ()  [unwired: 1 in, 1 out]
                n260 = shared-variable "Chan's target\\EtherCAT Master\\Device\\Motion Control-SetPoint"(w718) -> ()  [unwired: 1 in, 1 out]
              }
              frame "Dragging" {
                n261 = disable-structure shown="Enabled" {
                  disable-tunnel: w733 -> [_ w790]
                  frame Disabled {
                    # "Failed!\nYou should compensate the bias caued by gravity first."
                    # "Admittance Control by toques of each axis."
                    n262 = local read "Joint Vel"() -> (w762:T3)
                    n263 = local read "Torque Ratio"() -> (w761:T3)
                    n264 = Unbundle By Name(w762) -> ("Joint 1"=w756:sgl)
                    n265 = local read "Position"() -> (w767:T1)
                    n266 = Cluster To Array(cluster=w761) -> (array=w758:sgl[])
                    n267 = Equal To 0?(x=w756) -> (x = 0?=w753:bool)
                    n268 = local read "Joints(degree)"() -> (w769:T3)
                    n269 = Unbundle By Name(w761) -> ("Joint 1"=w763:sgl)
                    n270 = feedback #4(w758) -> (w759:sgl[])
                    n271 = Select(t=w758, s=w753, f=w759) -> (s? t:f=w760:sgl[])
                    n272 = feedback-in #4(w760) -> ()
                    n273 = Cluster To Array(cluster=w767) -> (array=w766:sgl[])
                    n274 = disable-structure shown="Enabled" {
                      disable-tunnel: [w775 w782] -> w752
                      disable-tunnel: w763 -> [w772 w778]
                      disable-tunnel: 2.0 ("x") -> [w770 w779]
                      disable-tunnel: [_ w777] -> w750
                      frame Disabled {
                        n275 = Subtract(x=w770, y=w772) -> (x-y=w776:dbl)
                        n276 = Sign(1:w776) -> (0:w774:dbl)
                        n277 = Absolute Value(x=w776) -> (abs(x)=w771:dbl)
                        n278 = Compound Arithmetic op=MULTIPLY("Kp", w771, w774) -> (w775:dbl)
                      }
                      frame Enabled {
                        n279 = Subtract(x=w779, y=w778) -> (x-y=w777:dbl)
                        n280 = call "PID r-y windup.vi"("Saturation"="Saturation", "PID Gains"="PID Gains", "Reference -\nEncoder position"=w777) -> ("Duty cycle"=w782:dbl)  [unwired: 5 in, 3 out]
                      }
                    }
                    n281 = Index Array(array=w760) -> ()  [unwired: 1 in, 1 out]
                    n282 = Cluster To Array(cluster=w769) -> (array=w768:sgl[])
                    n283 = local write "Pos"(w766) -> ()
                    n284 = local write "Joints"(w768) -> ()
                    n285 = Add(x="threshold", y=3.0) -> (x+y=w755:dbl)
                    n286 = Absolute Value(x=w750) -> (abs(x)=w751:dbl)
                    n287 = Select(t="threshold", s=w753, f=w755) -> (s? t:f=w747:dbl)
                    n288 = Greater?(x=w751, y=w747) -> (0:w749:bool)
                    n289 = disable-structure shown="Enabled" {
                      disable-tunnel: [w787 w788] -> w739
                      disable-tunnel: w751 -> [w785 _]
                      disable-tunnel: _ -> [w783 _]
                      disable-tunnel: w749 -> [_ w788]
                      frame Disabled {
                        n290 = feedback #5(w785) -> (w786:dbl)
                        n291 = feedback-in #5(w785) -> ()
                        n292 = Greater?(x=w785, y=w786) -> (0:w784:bool)
                        n293 = And(x=w784, y=w783) -> (x .and. y?=w787:bool)
                      }
                      frame Enabled {
                      }
                    }
                    n294 = Replace Array Subset(array=sgl[] [0.0, 0.0, 0.0, 0.0, 0.0, 0.0] ("Position"), new element=w752, index=0) -> (w740:sgl[])
                    n295 = Index Array(array=w740) -> (element #1=w741:sgl, element #2=w742:sgl, element #3=w743:sgl, element #4=w744:sgl, element #5=w745:sgl, element #6=w746:sgl)  [unwired: 6 in]
                    n296 = shared-variable "Chan's target\\EtherCAT Master\\Device\\Motion Control-SetPoint"(w739) -> ()  [unwired: 1 in, 1 out]
                    n297 = shared-variable "Chan's target\\EtherCAT Master\\Device\\Move-Move Command"(Commmands."MovejointsVel" ("Enum")) -> ()  [unwired: 1 in, 1 out]
                    n298 = shared-variable "Chan's target\\EtherCAT Master\\Device\\Move-SubIndex 001"(w741) -> ()  [unwired: 1 in, 1 out]
                    n299 = shared-variable "Chan's target\\EtherCAT Master\\Device\\Move-SubIndex 002"(w742) -> ()  [unwired: 1 in, 1 out]
                    n300 = shared-variable "Chan's target\\EtherCAT Master\\Device\\Move-SubIndex 003"(w743) -> ()  [unwired: 1 in, 1 out]
                    n301 = shared-variable "Chan's target\\EtherCAT Master\\Device\\Move-SubIndex 004"(w744) -> ()  [unwired: 1 in, 1 out]
                    n302 = shared-variable "Chan's target\\EtherCAT Master\\Device\\Move-SubIndex 005"(w745) -> ()  [unwired: 1 in, 1 out]
                    n303 = shared-variable "Chan's target\\EtherCAT Master\\Device\\Move-SubIndex 006"(w746) -> ()  [unwired: 1 in, 1 out]
                  }
                  frame Enabled {
                    # "Admittance Control by ATI sensor."
                    n304 = case shown="False" w790 {
                      frame False {
                        n305 = case shown="True" "Drag" {
                          frame False {
                            n306 = case shown="\"Short file\"" "TCP" {
                              frame "Long file", Default {
                                n307 = call "TCP.vi"("Save points"="Long", "find"="Search_Long") -> ("Record?"=→"Record":bool[], "TCP"=w796:sgl[])  [unwired: 4 out]
                                n308 = case shown="True" "Search_Long" {
                                tunnel: w796 -> [_ w797]
                                frame False {
                                }
                                frame True {
                                n309 = local read "SetTRF"() -> (w798:sgl[])
                                n310 = Replace Array Subset(array=w798, new element=w797) -> (w799:sgl[])  [unwired: 1 in]
                                n311 = local write "SetTRF"(w799) -> ()
                                }
                                }
                              }
                              frame "Short file" {
                                n312 = call "TCP.vi"("Save points"="Short", "find"="Search_Rotation") -> ("Record?"=→"Record":bool[], "TCP"=w803:sgl[])  [unwired: 4 out]
                                n313 = case shown="True" "Search_Rotation" {
                                tunnel: w803 -> [_ w804]
                                frame False {
                                }
                                frame True {
                                # "Target vector = long - short"
                                n314 = local read "SetTRF"() -> (w811:sgl[])
                                n315 = Array Subset(array=w811, index=0, length=3) -> (w806:sgl[])
                                n316 = Subtract(x=w806, y=w804) -> (x-y=w805:sgl[])
                                n317 = call "Vector to Euler angle.vi"("A Vector"=w805) -> ("alpha"=w809:sgl, "beta"=w808:sgl)
                                n318 = Replace Array Subset(array=w811, new element #1=w809, index #1=3 ("index"), new element #2=w808, index #2=4 ("index")) -> (w807:sgl[])
                                n319 = local write "SetTRF"(w807) -> ()
                                }
                                }
                              }
                            }
                          }
                          frame True {
                            n320 = local read "Adm_joints"() -> (w816:dbl[])
                            n321 = call "Is Value Changed.vim"("value"=w816) -> ("changed or first call?"=w815:bool)
                            n322 = case shown="True" w815 {
                              tunnel: w816 -> [_ w817]
                              frame False {
                              }
                              frame True {
                                n323 = call "Move-Move Command.vi"("Move-SubIndex"=w817, "Move-Move Command"=Commmands."Movejoints" ("Enum")) -> ()  [unwired: 1 in]
                              }
                            }
                          }
                        }
                      }
                      frame True {
                        n324 = local write "Drag"(FALSE ("Drag")) -> ()
                      }
                    }
                    n325 = local read "Position"() -> (→"Position":T1)
                  }
                }
                n326 = First Call?() -> (First Call?: T/F=w729:bool)
                n327 = Not(x=w729) -> (.not. x?=w730:bool)
                n328 = call "Is Value Changed.vim"("value"="Autotune") -> ("changed or first call?"=w731:bool)
                n329 = And(x=w730, y=w731) -> (x .and. y?=w732:bool)
                n330 = case shown="True" w732 {
                  frame False {
                  }
                  frame True {
                    n331 = local write "Waiting"(TRUE ("Homing")) -> ()
                    n332 = local write "Flags"(enum16{"Intro", "Homing", "Autotune"}."Autotune" ("Flags")) -> ()
                  }
                }
                n333 = case shown="\"Dragging\"" "Mode" {
                  frame "Self-Alignment" {
                    n334 = local write "k"(200.0 ("k")) -> ()
                  }
                  frame "Dragging" {
                    n335 = local write "k"(1200.0 ("k")) -> ()
                  }
                  frame "Custom", Default {
                  }
                }
              }
              frame "Demo" {
                # "Demo subpage"
                n336 = case shown="False" w834 {
                  frame False {
                    # "Compensate before starting"
                    n337 = local read "Demo subpages"() -> (w850:T11)
                    n338 = call "Is Value Changed.vim"("value"=w850) -> ("changed or first call?"=w849:bool)
                    n339 = case shown="\"Step 3\"" w850 {
                      tunnel: w849 -> [_ _ w1050]
                      frame "Step 3" {
                        n340 = call "Is Value Changed.vim"("value"="Exp-Rep") -> ("changed or first call?"=w852:bool)
                        n341 = disable-structure shown="Enabled" {
                          disable-tunnel: "Exp-Rep" -> [_ w892 w970]
                          disable-tunnel: w852 -> [_ w893 w969]
                          frame Disabled {
                            # "Section mode"
                            n342 = flat-sequence {
                              frame #0 {
                                n343 = shared-variable "Chan's target\\EtherCAT Master\\Device\\Motion Status-FIFO Space"() -> (w858:u16)  [unwired: 1 in, 1 out]
                                n344 = local read "Motions"() -> (w862:dbl[][])
                                n345 = Array Size(array=w862) -> (size(s)=w863:i32[])
                                n346 = local read "Counter"() -> (w859:i32)
                                n347 = Index Array(array=w863) -> (element=w860:i32)  [unwired: 1 in]
                                n348 = Greater Or Equal?(x=w859, y=w860) -> (x >= y?=w856:bool)
                                n349 = Equal?(x=w858, y=u16 13000) -> (x = y?=w854:bool)
                                n350 = And(y=w856) -> (x .and. y?=w861:bool)  [unwired: 1 in]
                                n351 = And(x=w856, y=w854) -> (x .and. y?=w855:bool)
                                n352 = case shown="True" w861 {
                                tunnel: w855 -> [w864 _]
                                frame False {
                                n353 = case shown="True" w864 {
                                frame False {
                                }
                                frame True {
                                n354 = local read "Joints(degree)"() -> (w866:T3)
                                n355 = local read item#-1() -> (w867)
                                n356 = Cluster To Array(cluster=w866) -> (array=w865:sgl[])
                                n357 = local write item#-1(FALSE ("Record")) -> ()
                                n358 = local write item#-1(w865) -> ()
                                n359 = local write item#-1(w867) -> ()
                                }
                                }
                                }
                                frame True {
                                # "Exp  initialization"
                                n360 = local write "Inverse Count"(0 ("Inverse Count")) -> ()
                                n361 = local write "Page_Motor"(T22."OTR Ctrl" ("Motor")) -> ()
                                n362 = local write "Counter"(-1 ("flag")) -> ()
                                n363 = local write "Rotate"(TRUE ("Rotate")) -> ()
                                n364 = local write item#-1(TRUE ("Record")) -> ()
                                n365 = local write "wait"(1 ("wait")) -> ()
                                n366 = local write item#-1(TRUE ("Record")) -> ()
                                }
                                }
                              }
                              frame #1 {
                                # "Read a row each time"
                                n367 = local read "Motions"() -> (w879:dbl[][])
                                n368 = Increment(x="Counter") -> (x+1=w876:i32)
                                n369 = Index Array(array=w879, index (row)=w876) -> (element=w882:dbl[])  [unwired: 1 in]
                                n370 = local write "Counter"(w876) -> ()
                                n371 = Array Size(array=w879) -> (size(s)=w878:i32[])
                                n372 = Index Array(array=w878) -> (element=w877:i32)  [unwired: 1 in]
                                n373 = Greater?(x=w877, y=w876) -> (0:w880:bool)
                                n374 = case shown="True" w880 {
                                tunnel: w882 -> [_ w890]
                                frame False {
                                }
                                frame True {
                                n375 = Index Array(array=w890) -> (element #1=w891:dbl, element #2=w888:dbl, element #3=w887:dbl, element #4=w886:dbl, element #5=w885:dbl, element #6=w884:dbl, element #7=w883:dbl)  [unwired: 7 in]
                                n376 = shared-variable "Chan's target\\EtherCAT Master\\Device\\Move-Move Command"(w891) -> ()  [unwired: 1 in, 1 out]
                                n377 = shared-variable "Chan's target\\EtherCAT Master\\Device\\Move-SubIndex 001"(w888) -> ()  [unwired: 1 in, 1 out]
                                n378 = shared-variable "Chan's target\\EtherCAT Master\\Device\\Move-SubIndex 002"(w887) -> ()  [unwired: 1 in, 1 out]
                                n379 = shared-variable "Chan's target\\EtherCAT Master\\Device\\Move-SubIndex 003"(w886) -> ()  [unwired: 1 in, 1 out]
                                n380 = shared-variable "Chan's target\\EtherCAT Master\\Device\\Move-SubIndex 004"(w885) -> ()  [unwired: 1 in, 1 out]
                                n381 = shared-variable "Chan's target\\EtherCAT Master\\Device\\Move-SubIndex 005"(w884) -> ()  [unwired: 1 in, 1 out]
                                n382 = shared-variable "Chan's target\\EtherCAT Master\\Device\\Move-SubIndex 006"(w883) -> ()  [unwired: 1 in, 1 out]
                                n383 = shared-variable "Chan's target\\EtherCAT Master\\Device\\Motion Control-SetPoint"(TRUE ("Motion Control-SetPoint")) -> ()  [unwired: 1 in, 1 out]
                                }
                                }
                              }
                            }
                          }
                          frame Enabled {
                            # "Self-Alignment + Torque Control"
                            n384 = case shown="True" w892 {
                              tunnel: w893 -> [_ w909]
                              frame False {
                                w896 = FALSE ("Drag")
                                n385 = local write "Drag"(w896) -> ()
                                n386 = local write "F_des"(dbl[] [0.0, 0.0, 0.0, 0.0, 0.0, 0.0] ("F_des")) -> ()
                                n387 = local write "Rotate"(w896) -> ()
                                n388 = local write "Exp-Rep"(w896) -> ()
                                n389 = local write "k"(1200.0 ("k")) -> ()
                              }
                              frame True {
                                n390 = flat-sequence {
                                tunnel: w909 -> [w910]
                                frame #0 {
                                # "Record Initial point"
                                n391 = case shown="True" w910 {
                                frame False {
                                }
                                frame True {
                                n392 = local write "DIR4"(TRUE ("DIR4")) -> ()
                                n393 = local write "Drag"(TRUE ("DIR4")) -> ()
                                n394 = local write "Rotate"(TRUE ("Rotate")) -> ()
                                n395 = local write "k"(200.0 ("k")) -> ()
                                }
                                }
                                }
                                frame #1 {
                                n396 = disable-structure shown="Enabled" {
                                frame Disabled {
                                # "Go back with constant"
                                # "Check if it is still for 3 sec"
                                n397 = feedback #6(0) -> (w920:i32)
                                n398 = Increment(x=w920) -> (x+1=w921:i32)
                                n399 = feedback #7(TRUE) -> (w916:bool)
                                n400 = Select(t=0, s=w916, f=w921) -> (s? t:f=w918:i32)
                                n401 = Greater?(x=w918, y=1500) -> (0:w923:bool)
                                n402 = case shown="False" w923 {
                                tunnel: [w927 w933] -> w925
                                tunnel: w918 -> [w926 w935]
                                tunnel: [w926 w935] -> w917
                                frame True {
                                # "Go back for 1 sec"
                                n403 = Greater?(x=w926, y=2000) -> (0:w927:bool)
                                n404 = Replace Array Subset(array=dbl[] [0.0, 0.0, 0.0, 0.0, 0.0, 0.0], new element="Back_force", index=2) -> (w930:dbl[])
                                n405 = local write "F_des"(w930) -> ()
                                }
                                frame False {
                                # "Max: 1N"
                                n406 = call "PID r-y windup_chan.vi"("Saturation"=dbl[] [0.0, 1.0]) -> ("Duty cycle"=w934:dbl, "PID Gains"=w939:cluster{"Kp":dbl, "Kd":dbl, "Ki":dbl}, "Reference"=w940:dbl)  [unwired: 5 in, 3 out]
                                n407 = Not Equal To 0?(x=w934) -> (x != 0?=w933:bool)
                                n408 = Replace Array Subset(array=dbl[] [0.0, 0.0, 0.0, 0.0, 0.0, 0.0], new element=w934, index=2) -> (w938:dbl[])
                                n409 = local write "F_des"(w938) -> ()
                                }
                                }
                                n410 = feedback-in #6(w917) -> ()
                                n411 = feedback-in #7(w925) -> ()
                                }
                                frame Enabled {
                                w948 = T24 2 items=["1-norm"=1, "2-norm"=2, "Inf-norm"=3, "-Inf-norm"=4, "User Defined"=5] ("norm type")
                                n412 = local read "External force_{t}"() -> (w952:T2)
                                n413 = local read "Adm_joints"() -> (w944:dbl[])
                                n414 = call "Is Value Changed.vim"("value"=w944) -> ("changed or first call?"=w943:bool)
                                n415 = Unbundle By Name(w952) -> ("Fex"=w951:dbl, "Fey"=w950:dbl)
                                n416 = case shown="True" w943 {
                                tunnel: w944 -> [_ w953]
                                frame False {
                                }
                                frame True {
                                n417 = call "Move-Move Command.vi"("Move-SubIndex"=w953, "Move-Move Command"=Commmands."Movejoints" ("Enum")) -> ()  [unwired: 1 in]
                                }
                                }
                                n418 = Build Array(w951, w950) -> (w949:dbl[])
                                n419 = call-poly <vilib>:"Vector Norm.vi"("norm type"=w948, "Input Vector"=w949) -> ("norm"=w947:dbl)  [unwired: 8 in, 1 out]
                                n420 = Less?(x=w947, y=1.0) -> (x < y?=w945:bool)
                                n421 = case shown="True" w945 {
                                tunnel: 100.0 ("k") -> [w957 w959]
                                frame False {
                                n422 = Multiply(x=w957, y=2.0) -> (x*y=w956:dbl)
                                n423 = local write "k"(w956) -> ()
                                n424 = local write "F_des"(dbl[] [0.0, 0.0, 0.0, 0.0, 0.0, 0.0] ("array")) -> ()
                                }
                                frame True {
                                # "Max: 1N"
                                n425 = local write "k"(w959) -> ()
                                n426 = local read "Torque (mNm)"() -> (w963:dbl)
                                n427 = Subtract(x="Torque_des", y=w963) -> (x-y=w961:dbl)
                                n428 = call "PID r-y windup.vi"("Saturation"="Saturation", "PID Gains"="PID_File feedrate", "Reference -\nEncoder position"=w961) -> ("Duty cycle"=w966:dbl)  [unwired: 5 in, 3 out]
                                n429 = Replace Array Subset(array=dbl[] [0.0, 0.0, 0.0, 0.0, 0.0, 0.0], new element=w966, index=2) -> (w965:dbl[])
                                n430 = local write "F_des"(w965) -> ()
                                }
                                }
                                }
                                }
                                }
                                }
                                n431 = call "Is Value Changed.vim"("value"="Compemsation") -> ("changed or first call?"=w908:bool)
                                n432 = And(x="Compemsation", y=w908) -> (x .and. y?=w906:bool)
                                n433 = local write "Add"(w906) -> ()
                                n434 = local read "Torque_des"() -> (w903:dbl)
                                n435 = local read "Saturation"() -> (w899:dbl[])
                                n436 = Subtract(x=w903, y="T_avg") -> (x-y=w901:dbl)
                                n437 = Index Array(array=w899, index=1) -> (element=w897:dbl)
                                n438 = Divide(x=w897, y=w901) -> (x/y=w900:dbl)
                                n439 = Bundle By Name(cluster=cluster{"Kp":dbl, "Kd":dbl, "Ki":dbl} {"Kp"=0.0, "Kd"=0.0, "Ki"=0.0} ("PID_File feedrate"), "Kp"=w900) -> (w904:cluster{"Kp":dbl, "Kd":dbl, "Ki":dbl})
                                n440 = local write "PID_File feedrate"(w904) -> ()
                              }
                            }
                          }
                          frame Disabled {
                            # "Only Self-Alignment"
                            n441 = case shown="True" w970 {
                              tunnel: w969 -> [_ w972]
                              frame False {
                                n442 = local write "Rotate"(FALSE ("Rotate")) -> ()
                              }
                              frame True {
                                n443 = flat-sequence {
                                tunnel: w972 -> [w974]
                                tunnel: [w974] -> w973
                                tunnel: w973 -> [w989]
                                frame #0 {
                                # "Record Initial point"
                                n444 = case shown="True" w974 {
                                frame False {
                                }
                                frame True {
                                (unwired) dbl[] [0.10000000000000003, 0.10000000000000003, 0.10000000000000003, 0.03, 0.03, 0.15000000000000002] ("Bi")
                                # "high sensitivity\nfor exp"
                                n445 = local read "Position"() -> (→"Start Points 2":T1)
                                n446 = local write "Rotate"(TRUE ("Rotate")) -> ()
                                n447 = local write "Bi"("Bi 3") -> ()
                                n448 = local write "k"(120.0 ("k")) -> ()
                                }
                                }
                                }
                                frame #1 {
                                # "Add counter one\nif satisfying case structure"
                                # "Initialize counter\nif restarting exp"
                                n449 = global read "Demo_forces.vi" "Fz"() -> (w995:dbl[])
                                n450 = Array Size(array=w995) -> (size(s)=w997:i32)
                                n451 = local read "Start Points 2"() -> (w1008:T1)
                                n452 = local read "Position"() -> (w984:T1)
                                n453 = Cluster To Array(cluster=w984) -> (array=w982:sgl[])
                                n454 = Cluster To Array(cluster=w1008) -> (array=w980:sgl[])
                                n455 = feedback #8(dbl[] [0.0, 0.0, 0.0, 0.0, 0.0, 0.0]) -> (w993:dbl[])
                                n456 = Array Subset(array=w982, length=3) -> (w981:sgl[])  [unwired: 1 in]
                                n457 = Array Subset(array=w980, length=3) -> (w979:sgl[])  [unwired: 1 in]
                                n458 = local read "Root length"() -> (w1005:dbl)
                                n459 = Subtract(x=w981, y=w979) -> (x-y=w1007:sgl[])
                                n460 = call-poly <vilib>:"Vector Norm.vi"("Input Vector"=w1007) -> ("norm"=w1006:dbl)  [unwired: 9 in, 1 out]
                                n461 = feedback #9(0) -> (w986:i32)
                                n462 = Select(t=0, s=w989, f=w986) -> (s? t:f=w987:i32)
                                n463 = Quotient & Remainder(x=w987, y=w997) -> (x-y*floor(x/y)=w996:i32)  [unwired: 1 out]
                                n464 = Index Array(array=w995, index=w996) -> (element=w991:dbl)
                                n465 = call "Is Value Changed.vim"("value"=w991) -> ("changed or first call?"=w998:bool)
                                n466 = Greater Than 0?(x=w991) -> (x > 0?=w1000:bool)
                                n467 = case shown="True" w1000 {
                                tunnel: [w1017 w1022] -> w999
                                tunnel: w998 -> [w1015 w1018]
                                frame False {
                                # "Initialize counter \nto zero."
                                # "Go back for 1.5 sec"
                                n468 = local write "DIR4"(FALSE ("DIR4")) -> ()
                                n469 = feedback #10(0) -> (w1012:i32)
                                n470 = Increment(x=w1012) -> (x+1=w1011:i32)
                                n471 = Select(t=0 ("Conter 3"), s=w1015, f=w1011) -> (s? t:f=w1010:i32)
                                n472 = feedback-in #10(w1010) -> ()
                                n473 = Equal?(x=w1010, y=750) -> (x = y?=w1017:bool)
                                }
                                frame True {
                                # "Go forth until being still for 2 sec"
                                n474 = local read "Position"() -> (w1029:T1)
                                n475 = local write "DIR4"(TRUE ("DIR4")) -> ()
                                n476 = call "Is Value Changed.vim"("value"=w1029) -> ("changed or first call?"=w1019:bool)
                                n477 = Or(x=w1018, y=w1019) -> (x .or. y?=w1020:bool)
                                n478 = feedback #11(0) -> (w1028:i32)
                                n479 = Increment(x=w1028) -> (x+1=w1026:i32)
                                n480 = Select(t=0, s=w1020, f=w1026) -> (s? t:f=w1024:i32)
                                n481 = feedback-in #11(w1024) -> ()
                                n482 = Equal?(x=w1024, y=1000) -> (x = y?=w1022:bool)
                                }
                                }
                                n483 = Replace Array Subset(array=w993, new element=w991, index=2) -> (w994:dbl[])
                                n484 = feedback-in #8(w994) -> ()
                                n485 = local write "F_des"(w994) -> ()
                                n486 = Increment(x=w987) -> (x+1=w1003:i32)
                                n487 = Less?(x=w1006, y=w1005) -> (x < y?=w1004:bool)
                                n488 = Select(t=w1003, s=w999, f=w987) -> (s? t:f=w1002:i32)
                                n489 = feedback-in #9(w1002) -> ()
                                n490 = case shown="False" w1004 {
                                frame False {
                                w1032 = FALSE ("Drag")
                                n491 = local write "Drag"(w1032) -> ()
                                n492 = local write "Rotate"(w1032) -> ()
                                n493 = local write "Exp-Rep"(w1032) -> ()
                                n494 = local write "k"(1200.0 ("k")) -> ()
                                n495 = local write "F_des"(dbl[] [0.0, 0.0, 0.0, 0.0, 0.0, 0.0] ("F_des")) -> ()
                                }
                                frame True {
                                n496 = local read "Adm_joints"() -> (w1034:dbl[])
                                n497 = local write "Drag"(TRUE ("Drag")) -> ()
                                n498 = call "Is Value Changed.vim"("value"=w1034) -> ("changed or first call?"=w1035:bool)
                                n499 = case shown="True" w1035 {
                                tunnel: w1034 -> [_ w1036]
                                frame False {
                                # "Stop joints and refresh adm parameters\nIf one of joints is over limit"
                                }
                                frame True {
                                n500 = Index Array(array=w1036) -> (element #1=w1043:dbl, element #2=w1042:dbl, element #3=w1041:dbl, element #4=w1040:dbl, element #5=w1039:dbl, element #6=w1038:dbl)  [unwired: 6 in]
                                n501 = shared-variable "Chan's target\\EtherCAT Master\\Device\\Move-Move Command"(Commmands."Movejoints" ("Enum")) -> ()  [unwired: 1 in, 1 out]
                                n502 = shared-variable "Chan's target\\EtherCAT Master\\Device\\Move-SubIndex 001"(w1043) -> ()  [unwired: 1 in, 1 out]
                                n503 = shared-variable "Chan's target\\EtherCAT Master\\Device\\Move-SubIndex 002"(w1042) -> ()  [unwired: 1 in, 1 out]
                                n504 = shared-variable "Chan's target\\EtherCAT Master\\Device\\Move-SubIndex 003"(w1041) -> ()  [unwired: 1 in, 1 out]
                                n505 = shared-variable "Chan's target\\EtherCAT Master\\Device\\Move-SubIndex 004"(w1040) -> ()  [unwired: 1 in, 1 out]
                                n506 = shared-variable "Chan's target\\EtherCAT Master\\Device\\Move-SubIndex 005"(w1039) -> ()  [unwired: 1 in, 1 out]
                                n507 = shared-variable "Chan's target\\EtherCAT Master\\Device\\Move-SubIndex 006"(w1038) -> ()  [unwired: 1 in, 1 out]
                                n508 = shared-variable "Chan's target\\EtherCAT Master\\Device\\Motion Control-SetPoint"(TRUE ("Motion Control-SetPoint")) -> ()  [unwired: 1 in, 1 out]
                                }
                                }
                                }
                                }
                                }
                                }
                              }
                            }
                          }
                        }
                      }
                      frame "Intro", Default {
                      }
                      frame "Step 1" {
                        # "Doctor Dragging Mode"
                        n509 = call "Is Value Changed.vim"("value"="Done") -> ("changed or first call?"=w1047:bool)
                        n510 = Not(x="Done") -> (.not. x?=w1048:bool)
                        n511 = And(x=w1048, y=w1047) -> (x .and. y?=w1045:bool)
                        n512 = Or(x=w1045, y=w1050) -> (x .or. y?=w1046:bool)
                        n513 = case shown="False" w1046 {
                          tunnel: "Done" -> [w1051 _]
                          frame False {
                            n514 = case shown="True" w1051 {
                              frame False {
                                n515 = local read "Adm_joints"() -> (w1053:dbl[])
                                n516 = local write "Drag"(TRUE ("Drag")) -> ()
                                n517 = call "Is Value Changed.vim"("value"=w1053) -> ("changed or first call?"=w1052:bool)
                                n518 = case shown="True" w1052 {
                                tunnel: w1053 -> [_ w1055]
                                frame False {
                                }
                                frame True {
                                n519 = call "Move-Move Command.vi"("Move-SubIndex"=w1055, "Move-Move Command"=Commmands."Movejoints" ("Enum")) -> ()  [unwired: 1 in]
                                }
                                }
                              }
                              frame True {
                                w1058 = sgl[] [79.370895, -0.46751443, 77.955, 1.2242525, -1.8750256, 0.0] ("SetTRF")
                                # "Self-Alignment Mode: Change sensor reference frame to tooltip"
                                n520 = local write "Drag"(FALSE ("Drag")) -> ()
                                n521 = local write "SetTRF"(w1058) -> ()
                                n522 = local write "Bi"(dbl[] [80.0, 80.0, 80.0, 80.0, 80.0, 80.0] ("Bi")) -> ()
                                n523 = Index Array(array=w1058) -> (element #1=w1065:sgl, element #2=w1064:sgl, element #3=w1063:sgl, element #4=w1062:sgl, element #5=w1061:sgl, element #6=w1060:sgl)  [unwired: 6 in]
                                n524 = shared-variable "Chan's target\\EtherCAT Master\\Device\\Move-Move Command"(Commmands."SetTRF" ("Enum")) -> ()  [unwired: 1 in, 1 out]
                                n525 = shared-variable "Chan's target\\EtherCAT Master\\Device\\Move-SubIndex 001"(w1065) -> ()  [unwired: 1 in, 1 out]
                                n526 = shared-variable "Chan's target\\EtherCAT Master\\Device\\Move-SubIndex 002"(w1064) -> ()  [unwired: 1 in, 1 out]
                                n527 = shared-variable "Chan's target\\EtherCAT Master\\Device\\Move-SubIndex 003"(w1063) -> ()  [unwired: 1 in, 1 out]
                                n528 = shared-variable "Chan's target\\EtherCAT Master\\Device\\Move-SubIndex 004"(w1062) -> ()  [unwired: 1 in, 1 out]
                                n529 = shared-variable "Chan's target\\EtherCAT Master\\Device\\Move-SubIndex 005"(w1061) -> ()  [unwired: 1 in, 1 out]
                                n530 = shared-variable "Chan's target\\EtherCAT Master\\Device\\Move-SubIndex 006"(w1060) -> ()  [unwired: 1 in, 1 out]
                                n531 = shared-variable "Chan's target\\EtherCAT Master\\Device\\Motion Control-SetPoint"(TRUE ("Motion Control-SetPoint")) -> ()  [unwired: 1 in, 1 out]
                              }
                            }
                          }
                          frame True {
                            w1068 = dbl[] [0.0, 0.0, 44.0, 0.0, 0.0, 0.0] ("Adm_joints")
                            # "This case is activated  when changing page or turning on \"Done\""
                            # "Doctor Dragging Mode: Change sensor reference frame to motor"
                            n532 = local write "F_des"(dbl[] [0.0, 0.0, 0.0, 0.0, 0.0, 0.0] ("Adm_joints")) -> ()
                            n533 = local write "Bi"(dbl[] [80.0, 80.0, 80.0, 160.0, 160.0, 160.0] ("Bi")) -> ()
                            n534 = local write "k"(1200.0 ("k")) -> ()
                            n535 = local write "SetTRF"(w1068) -> ()
                            n536 = call "Move-Move Command.vi"("Move-SubIndex"=w1068, "Move-Move Command"=Commmands."SetTRF" ("Enum")) -> ()  [unwired: 1 in]
                          }
                        }
                      }
                    }
                    n537 = case shown="True" w849 {
                      frame False {
                      }
                      frame True {
                        n538 = local write "Drag"(FALSE ("Drag")) -> ()
                      }
                    }
                  }
                  frame True {
                    n539 = local write "Intro"(TRUE ("Intro")) -> ()
                  }
                }
                n540 = Build Array("Intro", "Step1", "Step2", "Step3", "Setting") -> (w826:bool[])
                n541 = Array Size(array=w826) -> (size(s)=w831:i32)
                n542 = Initialize Array(FALSE, w831) -> (w830:bool[])
                n543 = feedback #12(w830) -> (w827:bool[])
                n544 = Exclusive Or(1:w827, 2:w826) -> (0:w828:bool[])
                n545 = Or Array Elements(Boolean array=w828) -> (logical OR=w829:bool)
                n546 = case shown="True" w829 {
                  tunnel: [w840 w847] -> w833
                  tunnel: w827 -> [w840 _]
                  tunnel: w828 -> [_ w847]
                  frame False {
                    # "Detect whether the page array is changed\nby using \"Array or\".\n\nOn top of that, By  using  \"exclusive or\",\nwe can get which slot is changed and\nreset the page array."
                  }
                  frame True {
                    n547 = Search 1D Array(1D array=w847, element=TRUE) -> (index of element=→"Demo subpages":i32)  [unwired: 1 in]
                    n548 = Index Array(array=w847) -> (element #1=w845:bool, element #2=w844:bool, element #3=w843:bool, element #4=w842:bool, element #5=w841:bool)  [unwired: 5 in]
                    n549 = local write "Intro"(w845) -> ()
                    n550 = local write "Step1"(w844) -> ()
                    n551 = local write "Step2"(w843) -> ()
                    n552 = local write "Step3"(w842) -> ()
                    n553 = local write "Setting"(w841) -> ()
                  }
                }
                n554 = feedback-in #12(w833) -> ()
                n555 = case shown="True" "Count avg" {
                  frame False {
                  }
                  frame True {
                    n556 = local read "Torque (mNm)"() -> (w838:dbl)
                    n557 = call "K avg filter (using FIR vi).vi"("avg num"=10, "x"=w838) -> ("Filtered x"=w837:dbl)  [unwired: 9 in]
                    n558 = local write "T_avg"(w837) -> ()
                    n559 = Add(x=w837, y=30.0) -> (x+y=w836:dbl)
                    n560 = local write "Torque_des"(w836) -> ()
                  }
                }
              }
              frame "Setting" {
                # "use exclusive or to check value change,\nif the changed value and its former data \nis oppsite sign, it will be -1."
                # "15"
                # "13"
                # "14"
                # "Send commands only when values change"
                # "7.16.24"
                # "8.9"
                # "10.11.12"
                n561 = Cluster To Array(cluster="Setting_Cart") -> (array=w1096:sgl[])
                n562 = Cluster To Array(cluster="Setting_Joints") -> (array=w1095:sgl[])
                n563 = Cluster To Array(cluster="Setting_Others") -> (array=w1094:sgl[])
                n564 = Build Array (concatenate)("SetWRF", "SetTRF") -> (w1088:sgl[])
                n565 = Build Array (concatenate)(w1096, w1095, w1094) -> (w1078:sgl[])
                n566 = feedback #13(w1088) -> (w1089:sgl[])
                n567 = feedback-in #13(w1088) -> ()
                n568 = call "Is Value Changed.vim"("value"=w1088) -> ("changed or first call?"=w1087:bool)
                n569 = Exclusive Or(1:w1089, 2:w1088) -> (0:w1091:i32[])
                n570 = feedback #14(w1078) -> (w1081:sgl[])
                n571 = feedback-in #14(w1078) -> ()
                n572 = Sign(1:w1091) -> (0:w1090:i32[])
                n573 = call "Is Value Changed.vim"("value"=w1078) -> ("changed or first call?"=w1082:bool)
                n574 = Exclusive Or(1:w1081, 2:w1078) -> (0:w1079:i32[])
                n575 = Absolute Value(x=w1090) -> (abs(x)=w1086:i32[])
                n576 = Sign(1:w1079) -> (0:w1080:i32[])
                n577 = case shown="True" w1087 {
                  tunnel: w1086 -> [_ w1123]
                  tunnel: "SetWRF" -> [_ w1116]
                  tunnel: "SetTRF" -> [_ w1117]
                  frame False {
                  }
                  frame True {
                    n578 = Search 1D Array(1D array=w1123, element=1) -> (index of element=w1121:i32)  [unwired: 1 in]
                    n579 = Less?(x=w1121, y=6) -> (x < y?=w1118:bool)
                    n580 = Select(t=w1116, s=w1118, f=w1117) -> (s? t:f=w1113:sgl[])
                    n581 = Select(t=u32 14 ("Move-Move Command"), s=w1118, f=u32 13 ("Move-Move Command")) -> (s? t:f=w1114:u32)
                    n582 = call "Move-Move Command.vi"("Move-SubIndex"=w1113, "Move-Move Command"=w1114) -> ()  [unwired: 1 in]
                  }
                }
                n583 = Absolute Value(x=w1080) -> (abs(x)=w1083:i32[])
                n584 = case shown="True" w1082 {
                  tunnel: w1083 -> [_ w1111]
                  tunnel: w1078 -> [_ w1108]
                  frame False {
                  }
                  frame True {
                    n585 = Search 1D Array(1D array=w1111, element=1) -> (index of element=w1106:i32)  [unwired: 1 in]
                    n586 = Index Array(array=u32[] [10, 11, 12, 8, 9, 7, 16, 24], index=w1106) -> (element=w1109:u32)
                    n587 = Index Array(array=w1108, index=w1106) -> (element=w1107:sgl)
                    n588 = shared-variable "Chan's target\\EtherCAT Master\\Device\\Move-SubIndex 001"(w1107) -> ()  [unwired: 1 in, 1 out]
                    n589 = shared-variable "Chan's target\\EtherCAT Master\\Device\\Move-Move Command"(w1109) -> ()  [unwired: 1 in, 1 out]
                    n590 = shared-variable "Chan's target\\EtherCAT Master\\Device\\Motion Control-SetPoint"(TRUE ("Motion Control-SetPoint")) -> ()  [unwired: 1 in, 1 out]
                  }
                }
                n591 = call "Is Value Changed.vim"("value"="Motion Control") -> ("changed or first call?"=w1076:bool)
                n592 = call "Is Value Changed.vim"("value"="Sim Mode") -> ("changed or first call?"=w1074:bool)
                n593 = call "Is Value Changed.vim"("value"="SetConf") -> ("changed or first call?"=w1093:bool)
                n594 = case shown="True" w1093 {
                  tunnel: "SetConf" -> [_ w1128]
                  frame False {
                  }
                  frame True {
                    n595 = Index Array(array=w1128) -> (element #1=w1127:sgl, element #2=w1126:sgl, element #3=w1125:sgl)  [unwired: 3 in]
                    n596 = shared-variable "Chan's target\\EtherCAT Master\\Device\\Move-Move Command"(u32 15 ("Move-Move Command")) -> ()  [unwired: 1 in, 1 out]
                    n597 = shared-variable "Chan's target\\EtherCAT Master\\Device\\Move-SubIndex 001"(w1127) -> ()  [unwired: 1 in, 1 out]
                    n598 = shared-variable "Chan's target\\EtherCAT Master\\Device\\Move-SubIndex 002"(w1126) -> ()  [unwired: 1 in, 1 out]
                    n599 = shared-variable "Chan's target\\EtherCAT Master\\Device\\Move-SubIndex 003"(w1125) -> ()  [unwired: 1 in, 1 out]
                    n600 = shared-variable "Chan's target\\EtherCAT Master\\Device\\Motion Control-SetPoint"(TRUE ("Motion Control-SetPoint")) -> ()  [unwired: 1 in, 1 out]
                  }
                }
                n601 = case shown="True" w1076 {
                  tunnel: "Motion Control" -> [_ w1101]
                  frame False {
                  }
                  frame True {
                    n602 = Unbundle By Name(w1101) -> ("Move ID"=w1102:u16, "Clear Move"=w1103:bool, "Reset PStop"=w1104:bool)
                    n603 = shared-variable "Chan's target\\EtherCAT Master\\Device\\Motion Control-Move ID"(w1102) -> ()  [unwired: 1 in, 1 out]
                    n604 = shared-variable "Chan's target\\EtherCAT Master\\Device\\Motion Control-Clear Move"(w1103) -> ()  [unwired: 1 in, 1 out]
                    n605 = shared-variable "Chan's target\\EtherCAT Master\\Device\\Motion Control-Reset PStop"(w1104) -> ()  [unwired: 1 in, 1 out]
                  }
                }
                n606 = case shown="True" w1074 {
                  tunnel: "Sim Mode" -> [_ w1100]
                  frame False {
                  }
                  frame True {
                    n607 = shared-variable "Chan's target\\EtherCAT Master\\Device\\Robot Control-Sim Mode"(w1100) -> ()  [unwired: 1 in, 1 out]
                  }
                }
              }
              frame "Waiting" {
                n608 = call "Is Value Changed.vim"("value"="Flags") -> ("changed or first call?"=w1130:bool)
                n609 = case shown="\"Autotune\"" "Flags" {
                  tunnel: w1130 -> [w1139 _ _]
                  frame "Autotune" {
                    w1133 = dbl[][] [[8.0, 5.0, 0.0, 0.0, 0.0, 0.0, 0.0], [1.0, 0.0, -30.0, 30.0, 90.0, 60.0, 100.0], [1.0, 0.0, -30.0, 30.0, -40.0, 10.0, 220.0], [1.0, 20.0, -20.0, 20.0, 0.0, 45.0, 170.0], [1.0, 0.0, -20.0, 20.0, 0.0, 30.0, 190.0], [1.0, 0.0, -20.0, 20.0, 45.0, 50.0, 190.0], [1.0, 10.0, -30.0, 40.0, 45.0, 40.0, 160.0], [1.0, 20.0, -30.0, 40.0, -45.0, 50.0, 150.0], [1.0, 0.0, -30.0, 30.0, 0.0, 60.0, 180.0], [8.0, 100.0, 0.0, 0.0, 0.0, 0.0, 0.0]]
                    # "Initialize counter"
                    # "read a row each time"
                    n610 = disable-structure shown="Disabled" {
                      disable-tunnel: [w1152 w1163] -> w1132
                      frame Disabled {
                        # "Not accurate"
                        # "Record data when Robot \nstaying a point for 0.3s"
                        # "Probe here and check \nhow many points you store"
                        n611 = shared-variable "Chan's target\\EtherCAT Master\\Device\\Motion Status-CheckPoint"() -> (w1149:u32)  [unwired: 1 in, 1 out]
                        n612 = call "Is Value Changed.vim"("value"=w1149) -> ("changed or first call?"=w1148:bool)
                        n613 = shared-variable "Chan's target\\EtherCAT Master\\Device\\Motion Status-EOB"() -> (w1151:bool)  [unwired: 1 in, 1 out]
                        n614 = feedback #15() -> (w1147:bool)  [unwired: 1 in]
                        n615 = feedback-in #15(w1148) -> ()
                        n616 = local write "Add"(w1147) -> ()
                        n617 = feedback #16(0) -> (w1157:i32)
                        n618 = Increment(x=w1157) -> (x+1=w1156:i32)
                        n619 = Select(t=w1156, s=w1147, f=w1157) -> (s? t:f=w1155:i32)
                        n620 = feedback-in #16(w1155) -> ()
                        n621 = feedback #17() -> (w1153:bool)  [unwired: 1 in]
                        n622 = feedback-in #17(w1151) -> ()
                        n623 = Equal?(x=w1149, y=u32 8) -> (x = y?=w1150:bool)
                        n624 = Compound Arithmetic op=AND(w1153, w1151, w1150) -> (w1152:bool)
                      }
                      frame Enabled {
                        w1159 = 0
                        # "Probe here and check \nhow many points you store"
                        # "Record data per 0.4 seconds to give\nCompensation.vi enough time to culculate."
                        n625 = shared-variable "Chan's target\\EtherCAT Master\\Device\\Motion Status-EOB"() -> (w1161:bool)  [unwired: 1 in, 1 out]
                        n626 = feedback #18(0) -> (w1170:i32)
                        n627 = Increment(x=w1170) -> (x+1=w1168:i32)
                        n628 = Quotient & Remainder(x=w1168, y=200) -> (x-y*floor(x/y)=w1167:i32)  [unwired: 1 out]
                        n629 = feedback-in #18(w1167) -> ()
                        n630 = Equal To 0?(x=w1167) -> (x = 0?=w1166:bool)
                        n631 = local write "Add"(w1166) -> ()
                        n632 = feedback #19(w1159) -> (w1160:i32)
                        n633 = Select(t=w1160, s=w1161, f=w1159) -> (s? t:f=w1165:i32)
                        n634 = feedback #20(0) -> (w1172:i32)
                        n635 = Increment(x=w1172) -> (x+1=w1173:i32)
                        n636 = Select(t=w1173, s=w1166, f=w1172) -> (s? t:f=w1174:i32)
                        n637 = feedback-in #20(w1174) -> ()
                        n638 = Increment(x=w1165) -> (x+1=w1162:i32)
                        n639 = feedback-in #19(w1162) -> ()
                        n640 = Equal?(x=w1162, y=200) -> (x = y?=w1163:bool)
                      }
                    }
                    n641 = Bundle By Name(cluster=cluster{"SetJointVel":sgl, "SetJointAcc":sgl} {"SetJointVel"=100.0, "SetJointAcc"=150.0} ("Setting_Joints"), "SetJointVel"=sgl 100.0) -> (w1142:cluster{"SetJointVel":sgl, "SetJointAcc":sgl})
                    n642 = feedback #21(-1) -> (w1136:i32)
                    n643 = Select(t=-1, s=w1139, f=w1136) -> (s? t:f=w1137:i32)
                    n644 = Increment(x=w1137) -> (x+1=w1135:i32)
                    n645 = feedback-in #21(w1135) -> ()
                    n646 = Index Array(array=w1133, index (row)=w1135) -> (element=w1146:dbl[])  [unwired: 1 in]
                    n647 = local write "Setting_Joints"(w1142) -> ()
                    n648 = Array Size(array=w1133) -> (size(s)=w1145:i32[])
                    n649 = Index Array(array=w1145) -> (element=w1144:i32)  [unwired: 1 in]
                    n650 = Greater?(x=w1144, y=w1135) -> (0:w1141:bool)
                    n651 = case shown="True" w1141 {
                      tunnel: w1146 -> [_ w1180]
                      frame False {
                      }
                      frame True {
                        n652 = Index Array(array=w1180) -> (element=w1178:dbl)  [unwired: 1 in]
                        n653 = Array Subset(array=w1180, index=1, length=6) -> (w1179:dbl[])
                        n654 = call "Move-Move Command.vi"("Move-SubIndex"=w1179, "Move-Move Command"=w1178) -> ()  [unwired: 1 in]
                      }
                    }
                    n655 = case shown="True" w1132 {
                      frame False {
                      }
                      frame True {
                        n656 = local write "Flags"(enum16{"Intro", "Homing", "Autotune"}."Intro" ("Flags")) -> ()
                        n657 = local write "Add"(FALSE ("Add")) -> ()
                      }
                    }
                  }
                  frame "Intro", Default {
                    n658 = shared-variable "Chan's target\\EtherCAT Master\\Device\\Robot Status-Homed"() -> (w1183:bool)  [unwired: 1 in, 1 out]
                    n659 = local write "Intro"(w1183) -> ()
                  }
                  frame "Homing" {
                    n660 = local write "Flags"(enum16{"Intro", "Homing", "Autotune"}."Intro" ("Flags")) -> ()
                    n661 = call "Move-Move Command.vi"("Move-SubIndex"=sgl[] [0.0, -30.0, 30.0, 0.0, 60.0, 180.0] ("Move SubIndex"), "Move-Move Command"=Commmands."Movejoints") -> ()  [unwired: 1 in]
                  }
                }
              }
              frame "Intro", Default {
                # "Do nothing and make this page be a default page"
              }
            }
          }
        }
        n662 = call "Delay count.vi"("Finished Late? [i-1]"=w658) -> ("Count"=→"Control loop":u32)
        n663 = call "Is Value Changed.vim"("value"="Pause") -> ("changed or first call?"=w654:bool)
        n664 = call "Is Value Changed.vim"("value"="Reset") -> ("changed or first call?"=w656:bool)
        n665 = case shown="True" w654 {
          tunnel: "Pause" -> [_ w1192]
          frame False {
          }
          frame True {
            n666 = shared-variable "Chan's target\\EtherCAT Master\\Device\\Motion Control-Pause"(w1192) -> ()  [unwired: 1 in, 1 out]
          }
        }
        n667 = case shown="True" w656 {
          tunnel: "Reset" -> [_ w1193]
          frame False {
          }
          frame True {
            n668 = shared-variable "Chan's target\\EtherCAT Master\\Device\\Robot Control-Reset Error"(w1193) -> ()  [unwired: 1 in, 1 out]
          }
        }
        n669 = First Call?() -> (First Call?: T/F=w649:bool)
        n670 = call "Is Value Changed.vim"("value"="Activate") -> ("changed or first call?"=w652:bool)
        n671 = Not(x=w649) -> (.not. x?=w648:bool)
        n672 = And(x=w648, y=w652) -> (x .and. y?=w650:bool)
        n673 = case shown="True" w650 {
          tunnel: "Activate" -> [_ w1190]
          frame False {
          }
          frame True {
            n674 = Not(x=w1190) -> (.not. x?=w1191:bool)
            n675 = shared-variable "Chan's target\\EtherCAT Master\\Device\\Robot Control-Activate"(w1190) -> ()  [unwired: 1 in, 1 out]
            n676 = shared-variable "Chan's target\\EtherCAT Master\\Device\\Robot Control-Home"(w1190) -> ()  [unwired: 1 in, 1 out]
            n677 = shared-variable "Chan's target\\EtherCAT Master\\Device\\Robot Control-Deactivate"(w1191) -> ()  [unwired: 1 in, 1 out]
            n678 = local write "Waiting"(TRUE ("Waiting")) -> ()
          }
        }
        n679 = First Call?() -> (First Call?: T/F=w645:bool)
        n680 = Not(x=w645) -> (.not. x?=w646:bool)
        n681 = call "Is Value Changed.vim"("value"="Home") -> ("changed or first call?"=w643:bool)
        n682 = And(x=w646, y=w643) -> (x .and. y?=w644:bool)
        n683 = case shown="True" w644 {
          frame False {
          }
          frame True {
            n684 = local write "Flags"(enum16{"Intro", "Homing", "Autotune"}."Homing" ("Flags")) -> ()
            n685 = local write "Waiting"(TRUE ("Homing")) -> ()
          }
        }
        n686 = local read "stop"() -> (w659:bool)
        n687 = node-c288() -> ()  [unwired: 1 in, 1 out]
      }
      n688 = timed-loop {
        timing: w142 -> [_]
        timing-out: [_] -> w141
        stop <- w308 stop-if-true
        # "ATI-mini40"
        n689 = node-c288() -> ()  [unwired: 1 in, 1 out]
        n690 = Scale By Power Of 2(n="Filter", x=u8 1) -> (x*2^n=w316:u8)
        n691 = Equal To 0?(x="Calibration") -> (x = 0?=w327:bool)
        n692 = Number To Boolean Array(number=w316) -> (Boolean array=w315:bool[])
        n693 = Initialize Array(FALSE, 32 ("dimension size")) -> (w323:bool[])
        n694 = Index Array(array=w315) -> (element #1=w314:bool, element #2=w313:bool, element #3=w312:bool, element #4=w311:bool)  [unwired: 4 in]
        n695 = Initialize Array(FALSE, 32 ("dimension size")) -> (w297:bool[])
        n696 = feedback #22(w323) -> (w329:bool[])
        n697 = Replace Array Subset(array=w329, new element #1="Zeroing", index #1=0 ("index"), new element #2=w327, index #2=8 ("index"), new element #3=w314, index #3=4 ("index"), new element #4=w313, index #4=5 ("index"), new element #5=w312, index #5=6 ("index"), new element #6=w311, index #6=7 ("index")) -> (w322:bool[])
        n698 = feedback-in #22(w322) -> ()
        n699 = feedback #23(w297) -> (w293:bool[])
        n700 = Replace Array Subset(array=w293, new element="Sensor Transform", index=19) -> (w298:bool[])
        n701 = feedback-in #23(w298) -> ()
        n702 = Boolean Array To Number(Boolean array=w322) -> (number=w291:u32)
        n703 = Boolean Array To Number(Boolean array=w298) -> (number=w289:u32)
        n704 = call "Is Value Changed.vim"("value"=w291) -> ("changed or first call?"=w292:bool)
        n705 = call "Is Value Changed.vim"("value"=w289) -> ("changed or first call?"=w290:bool)
        n706 = case shown="True" w292 {
          tunnel: w291 -> [_ w335]
          frame False {
          }
          frame True {
            n707 = shared-variable "Chan's target\\EtherCAT Master\\Device2\\Control Codes-Control 1"(w335) -> ()  [unwired: 1 in, 1 out]
          }
        }
        n708 = case shown="True" w290 {
          tunnel: w289 -> [_ w334]
          frame False {
          }
          frame True {
            n709 = shared-variable "Chan's target\\EtherCAT Master\\Device2\\Control Codes-Control 2"(w334) -> ()  [unwired: 1 in, 1 out]
          }
        }
        n710 = shared-variable "Chan's target\\EtherCAT Master\\Device2\\Reading Data-Status Code"() -> (w300:u32)  [unwired: 1 in, 1 out]
        n711 = shared-variable "Chan's target\\EtherCAT Master\\Device2\\Reading Data-Fx"() -> (w304:i32)  [unwired: 1 in, 1 out]
        n712 = shared-variable "Chan's target\\EtherCAT Master\\Device2\\Reading Data-Fy"() -> (w303:i32)  [unwired: 1 in, 1 out]
        n713 = shared-variable "Chan's target\\EtherCAT Master\\Device2\\Reading Data-Fz"() -> (w287:i32)  [unwired: 1 in, 1 out]
        n714 = shared-variable "Chan's target\\EtherCAT Master\\Device2\\Reading Data-Tx"() -> (w302:i32)  [unwired: 1 in, 1 out]
        n715 = shared-variable "Chan's target\\EtherCAT Master\\Device2\\Reading Data-Ty"() -> (w288:i32)  [unwired: 1 in, 1 out]
        n716 = shared-variable "Chan's target\\EtherCAT Master\\Device2\\Reading Data-Tz"() -> (w301:i32)  [unwired: 1 in, 1 out]
        n717 = Number To Boolean Array(number=w300) -> (Boolean array=w310:bool[])
        n718 = Bundle(w304, w303, w287, w302, w288, w301) -> (w333:cluster{i32, i32, i32, i32, i32, i32})  [unwired: 1 in]
        n719 = Index Array(array=w310, index=31) -> (element=→"Sensor_err":bool)
        n720 = local read "stop"() -> (w308:bool)
        n721 = Divide(x=w333, y=cluster{i32, i32, i32, i32, i32, i32} {1000000, 1000000, 1000000, 1000000, 1000000, 1000000}) -> (x/y=→"Sensor":cluster{dbl, dbl, dbl, dbl, dbl, dbl})
        n722 = node-c288() -> ()  [unwired: 1 in, 1 out]
      }
      n723 = timed-loop {
        timing: w152 -> [_]
        timing-out: [_] -> w151
        stop <- w631 stop-if-true
        w568 = 3 ("index")
        w578 = 3 ("index")
        # "Motor's position"
        # "Sensor Compensation"
        # "Note:\nOpening this subvi while \nit is running will delay UI."
        # "Acceleration"
        # "Joint Vel"
        # "Torque Ratio"
        # "Position Status"
        # "Joints Status"
        # "Motion Status"
        # "Robot Status"
        # "Meca500_Monitor"
        n724 = node-c288() -> (w595:bool)  [unwired: 1 in]
        n725 = shared-variable "Chan's target\\EtherCAT Master\\Device\\Robot Status-Error"() -> (w637:u16)  [unwired: 1 in, 1 out]
        "Error code" <- w637
        n726 = shared-variable "Chan's target\\EtherCAT Master\\Device\\Robot Status-Busy"() -> (w632:bool)  [unwired: 1 in, 1 out]
        n727 = shared-variable "Chan's target\\EtherCAT Master\\Device\\Robot Status-Activated"() -> (w633:bool)  [unwired: 1 in, 1 out]
        n728 = shared-variable "Chan's target\\EtherCAT Master\\Device\\Robot Status-Homed"() -> (w634:bool)  [unwired: 1 in, 1 out]
        n729 = shared-variable "Chan's target\\EtherCAT Master\\Device\\Robot Status-SimActivated"() -> (w635:bool)  [unwired: 1 in, 1 out]
        n730 = call "Delay count.vi"("Finished Late? [i-1]"=w595) -> ("Count"=→"Monitor loop":u32)
        n731 = Not Equal To 0?(x=w637) -> (x != 0?=w616:bool)
        n732 = Bundle(w616, w632, w633, w634, w635) -> (→"Robot Status":cluster{bool, bool, bool, bool, bool})  [unwired: 1 in]
        n733 = shared-variable "Chan's target\\EtherCAT Master\\Device\\Motion Status-Move ID"() -> (w625:u16)  [unwired: 1 in, 1 out]
        n734 = shared-variable "Chan's target\\EtherCAT Master\\Device\\Motion Status-FIFO Space"() -> (w626:u16)  [unwired: 1 in, 1 out]
        n735 = shared-variable "Chan's target\\EtherCAT Master\\Device\\Motion Status-Paused"() -> (w615:bool)  [unwired: 1 in, 1 out]
        n736 = shared-variable "Chan's target\\EtherCAT Master\\Device\\Motion Status-EOB"() -> (w627:bool)  [unwired: 1 in, 1 out]
        n737 = shared-variable "Chan's target\\EtherCAT Master\\Device\\Motion Status-EOM"() -> (w628:bool)  [unwired: 1 in, 1 out]
        n738 = shared-variable "Chan's target\\EtherCAT Master\\Device\\Motion Status-FIFO Cleared"() -> (w614:bool)  [unwired: 1 in, 1 out]
        n739 = shared-variable "Chan's target\\EtherCAT Master\\Device\\Motion Status-PStop"() -> (w629:bool)  [unwired: 1 in, 1 out]
        n740 = Bundle(w625, w626, w615, w627, w628, w614, w629) -> (→"Motion Status":cluster{u16, u16, bool, bool, bool, bool, bool})  [unwired: 1 in]
        n741 = shared-variable "Chan's target\\EtherCAT Master\\Device\\Joint Set-SubIndex 001"() -> (w587:sgl)  [unwired: 1 in, 1 out]
        n742 = shared-variable "Chan's target\\EtherCAT Master\\Device\\Joint Set-SubIndex 002"() -> (w586:sgl)  [unwired: 1 in, 1 out]
        n743 = shared-variable "Chan's target\\EtherCAT Master\\Device\\Joint Set-SubIndex 003"() -> (w585:sgl)  [unwired: 1 in, 1 out]
        n744 = shared-variable "Chan's target\\EtherCAT Master\\Device\\Joint Set-SubIndex 004"() -> (w582:sgl)  [unwired: 1 in, 1 out]
        n745 = shared-variable "Chan's target\\EtherCAT Master\\Device\\Joint Set-SubIndex 005"() -> (w583:sgl)  [unwired: 1 in, 1 out]
        n746 = shared-variable "Chan's target\\EtherCAT Master\\Device\\Joint Set-SubIndex 006"() -> (w584:sgl)  [unwired: 1 in, 1 out]
        n747 = Bundle(w587, w586, w585, w582, w583, w584) -> (→"Joints(degree)":cluster{sgl, sgl, sgl, sgl, sgl, sgl})  [unwired: 1 in]
        n748 = Build Array(w587, w586, w585, w582, w583, w584) -> (w590:sgl[])
        n749 = local read "Sensor"() -> (w589:T6)
        n750 = local read "Instance"() -> (w580:T7)
        n751 = local read "SetTRF"() -> (w581:sgl[])
        n752 = call "Sensor Compensation.vi"("Init"=w580, "Joints"=w590, "Sensor"=w589, "Add"="Add") -> ("Weight (g)"=→"Weight (g)":dbl, "theta(degree)"=→"theta(degree)":dbl, "Compensation"=w576:T2, "Record"=→"Instance":T7)
        "External force_{S}" <- w576
        n753 = call "Tool Transformation.vi"("SetTRF"=w581, "External force"=w576) -> ("Rotation Matrix"=→"Rt_S":dbl[][], "External force"=w567:T2)
        "External force_{t}" <- w567
        n754 = call "Tool Transformation.vi"("SetTRF"=sgl[] [24.0, 0.0, 48.0, 0.0, 0.0, 0.0], "External force"=w576) -> ("External force"=w575:T2)  [unwired: 1 out]
        n755 = Cluster To Array(cluster=w575) -> (array=w563:dbl[])
        n756 = Array Subset(array=w563, index=w578, length=w578) -> (w564:dbl[])
        n757 = Cluster To Array(cluster=w567) -> (array=w570:dbl[])
        n758 = Multiply(x=w564, y=1000.0) -> (x*y=w574:dbl[])
        n759 = global write "Sensor_m.vi" "Sensor_{m}"(w563) -> ()
        n760 = Array Subset(array=w570, index=w568, length=w568) -> (w569:dbl[])
        n761 = Multiply(x=w574, y=67) -> (x*y=→"Torque (mNm) 2":dbl[])
        n762 = Multiply(x=w569, y=1000.0) -> (x*y=→"x*y":dbl[])
        n763 = shared-variable "Chan's target\\EtherCAT Master\\Device\\End-Effector Pose-SubIndex 001"() -> (w618:sgl)  [unwired: 1 in, 1 out]
        n764 = shared-variable "Chan's target\\EtherCAT Master\\Device\\End-Effector Pose-SubIndex 002"() -> (w619:sgl)  [unwired: 1 in, 1 out]
        n765 = shared-variable "Chan's target\\EtherCAT Master\\Device\\End-Effector Pose-SubIndex 003"() -> (w620:sgl)  [unwired: 1 in, 1 out]
        n766 = shared-variable "Chan's target\\EtherCAT Master\\Device\\End-Effector Pose-SubIndex 004"() -> (w621:sgl)  [unwired: 1 in, 1 out]
        n767 = shared-variable "Chan's target\\EtherCAT Master\\Device\\End-Effector Pose-SubIndex 005"() -> (w622:sgl)  [unwired: 1 in, 1 out]
        n768 = shared-variable "Chan's target\\EtherCAT Master\\Device\\End-Effector Pose-SubIndex 006"() -> (w623:sgl)  [unwired: 1 in, 1 out]
        n769 = Bundle(w618, w619, w620, w621, w622, w623) -> (→"Position":cluster{sgl, sgl, sgl, sgl, sgl, sgl})  [unwired: 1 in]
        n770 = shared-variable "Chan's target\\EtherCAT Master\\Device\\Torque Ratio-SubIndex 001"() -> (w601:sgl)  [unwired: 1 in, 1 out]
        n771 = shared-variable "Chan's target\\EtherCAT Master\\Device\\Torque Ratio-SubIndex 002"() -> (w600:sgl)  [unwired: 1 in, 1 out]
        n772 = shared-variable "Chan's target\\EtherCAT Master\\Device\\Torque Ratio-SubIndex 003"() -> (w599:sgl)  [unwired: 1 in, 1 out]
        n773 = shared-variable "Chan's target\\EtherCAT Master\\Device\\Torque Ratio-SubIndex 004"() -> (w598:sgl)  [unwired: 1 in, 1 out]
        n774 = shared-variable "Chan's target\\EtherCAT Master\\Device\\Torque Ratio-SubIndex 005"() -> (w597:sgl)  [unwired: 1 in, 1 out]
        n775 = shared-variable "Chan's target\\EtherCAT Master\\Device\\Torque Ratio-SubIndex 006"() -> (w596:sgl)  [unwired: 1 in, 1 out]
        n776 = Bundle(w601, w600, w599, w598, w597, w596) -> (→"Torque Ratio":cluster{sgl, sgl, sgl, sgl, sgl, sgl})  [unwired: 1 in]
        n777 = shared-variable "Chan's target\\EtherCAT Master\\Device\\Joint velocities-SubIndex 001"() -> (w612:sgl)  [unwired: 1 in, 1 out]
        n778 = shared-variable "Chan's target\\EtherCAT Master\\Device\\Joint velocities-SubIndex 002"() -> (w611:sgl)  [unwired: 1 in, 1 out]
        n779 = shared-variable "Chan's target\\EtherCAT Master\\Device\\Joint velocities-SubIndex 003"() -> (w610:sgl)  [unwired: 1 in, 1 out]
        n780 = shared-variable "Chan's target\\EtherCAT Master\\Device\\Joint velocities-SubIndex 004"() -> (w609:sgl)  [unwired: 1 in, 1 out]
        n781 = shared-variable "Chan's target\\EtherCAT Master\\Device\\Joint velocities-SubIndex 005"() -> (w608:sgl)  [unwired: 1 in, 1 out]
        n782 = shared-variable "Chan's target\\EtherCAT Master\\Device\\Joint velocities-SubIndex 006"() -> (w607:sgl)  [unwired: 1 in, 1 out]
        n783 = Bundle(w612, w611, w610, w609, w608, w607) -> (→"Joint Vel":cluster{sgl, sgl, sgl, sgl, sgl, sgl})  [unwired: 1 in]
        n784 = shared-variable "Chan's target\\EtherCAT Master\\Device\\Accelerometer-X"() -> (w605:i32)  [unwired: 1 in, 1 out]
        n785 = shared-variable "Chan's target\\EtherCAT Master\\Device\\Accelerometer-Y"() -> (w604:i32)  [unwired: 1 in, 1 out]
        n786 = shared-variable "Chan's target\\EtherCAT Master\\Device\\Accelerometer-Z"() -> (w603:i32)  [unwired: 1 in, 1 out]
        n787 = Bundle(w605, w604, w603) -> (→"Acceration":cluster{i32, i32, i32})  [unwired: 1 in]
        n788 = local read "stop"() -> (w631:bool)
        n789 = node-c288() -> ()  [unwired: 1 in, 1 out]
      }
      n790 = timed-loop {
        timing: w148 -> [_]
        timing-out: [_] -> w147
        stop <- "stop" stop-if-true
        # "Current Detection"
        n791 = node-c288() -> ()  [unwired: 1 in, 1 out]
        n792 = local read "External force_{S}"() -> (w350:T2)
        n793 = local read "Torque (mNm)"() -> (w340:dbl)
        "Toqrues(plot)" <- w340
        n794 = global write "File_Torque.vi" "File_Torque (mNm)"(w340) -> ()
        n795 = Unbundle By Name(w350) -> ("Fex"=w345:dbl, "Fey"=w344:dbl, "Fez"=w343:dbl)
        n796 = Unbundle By Name(w350) -> ("£nex"=w349:dbl, "£ney"=w348:dbl, "£nez"=w347:dbl)
        n797 = Bundle("Fex"=w345, "Fey"=w344, "Fez"=w343) -> (→"Forces(plot)":cluster{"Fex":dbl, "Fey":dbl, "Fez":dbl})  [unwired: 1 in]
        n798 = Bundle("£nex"=w349, "£ney"=w348, "£nez"=w347) -> (→"Torques(plot)":cluster{" £nex":dbl, " £ney":dbl, " £nez":dbl})  [unwired: 1 in]
        n799 = node-c288() -> ()  [unwired: 1 in, 1 out]
      }
      n800 = while {
        stop <- w367 stop-if-true
        w375 = refnum<k21> refnum  # IndComECAT Slave
        # "Help btn"
        # "Connection status"
        # "Motion Control-Pause should be \nlinked with Motion Status-Paused"
        # "Progress bar"
        # "Errors"
        # "In this way, if there are multiple errors, \nit may show just one error"
        # "Pages"
        # "User Interface"
        n801 = Build Array("Joint Ctrl", "Pos Ctrl", "Jogging", "Dragging", "RCT", "Setting", "Intro", "Waiting") -> (w364:bool[])
        n802 = Array Size(array=w364) -> (size(s)=w363:i32)
        n803 = Initialize Array(FALSE, w363) -> (w365:bool[])
        n804 = feedback #24(w365) -> (w398:bool[])
        n805 = Exclusive Or(1:w398, 2:w364) -> (0:w397:bool[])
        n806 = Or Array Elements(Boolean array=w397) -> (logical OR=w369:bool)
        n807 = case shown="True" w369 {
          tunnel: [w451 w452] -> w395
          tunnel: w398 -> [w451 _]
          tunnel: w397 -> [_ w452]
          frame False {
            # "Detect whether the page array is changed\nby using \"Array or\".\n\nOn top of that, By  using  \"exclusive or\",\nwe can get which slot is changed and\nreset the page array."
          }
          frame True {
            n808 = Search 1D Array(1D array=w452, element=TRUE) -> (index of element=w454:i32)  [unwired: 1 in]
            n809 = Index Array(array=w452) -> (element #1=w462:bool, element #2=w461:bool, element #3=w460:bool, element #4=w459:bool, element #5=w458:bool, element #6=w457:bool, element #7=w456:bool, element #8=w455:bool)  [unwired: 8 in]
            n810 = local write "Joint Ctrl"(w462) -> ()
            n811 = local write "Pos Ctrl"(w461) -> ()
            n812 = local write "Jogging"(w460) -> ()
            n813 = local write "Dragging"(w459) -> ()
            n814 = local write "RCT"(w458) -> ()
            n815 = local write "Setting"(w457) -> ()
            n816 = local write "Intro"(w456) -> ()
            n817 = local write "Waiting"(w455) -> ()
            n818 = local write "Pages"(w454) -> ()
          }
        }
        n819 = feedback-in #24(w395) -> ()
        n820 = local read "Monitor loop"() -> (w393:u32)
        n821 = local read "Control loop"() -> (w394:u32)
        n822 = local read "Finished_late"() -> (w388:u32)
        n823 = local read "Error code"() -> (w391:u16)
        n824 = local read "Sensor_err"() -> (w362:bool)
        n825 = Not Equal To 0?(x=w388) -> (x != 0?=w387:bool)
        n826 = Not Equal To 0?(x=w394) -> (x != 0?=w386:bool)
        n827 = Not Equal To 0?(x=w393) -> (x != 0?=w392:bool)
        n828 = Not Equal To 0?(x=w391) -> (x != 0?=w380:bool)
        n829 = Build Array(w386, w392, w380, w387, w362) -> (w390:bool[])
        n830 = Search 1D Array(1D array=w390, element=TRUE ("Visible")) -> (index of element=w379:i32)  [unwired: 1 in]
        n831 = call "Is Value Changed.vim"("value"=w379) -> ("changed or first call?"=w378:bool)
        n832 = case shown="1" w379 {
          tunnel: w378 -> [w424 _ _ _ _ _]
          tunnel: ["Unknown" ("ERROR") "Finished late-\nControl loop" ("ERROR") "Finished late -\nMonitor loop" ("ERROR") w433 "Finished late-\nTool loop" ("ERROR") "F/T Sensor " ("ERROR")] -> w377
          frame -1, Default {
            # "item showd by property node-Visible should use property node-Value to change value."
            n833 = case shown="True" w424 {
              frame False {
              }
              frame True {
                w425 = FALSE ("Visible")
                n834 = property on="ERROR" class="Str"("Visible"=w425) -> ()  [unwired: 2 in, 2 out]
                n835 = property on="Reset" class="Bool"("Visible"=w425) -> ()  [unwired: 2 in, 2 out]
              }
            }
          }
          frame 0 {
            n836 = property on="ERROR" class="Str"("Visible"=TRUE) -> ()  [unwired: 2 in, 2 out]
          }
          frame 1 {
            n837 = property on="ERROR" class="Str"("Visible"=TRUE) -> ()  [unwired: 2 in, 2 out]
          }
          frame 2 {
            w436 = TRUE ("Visible")
            n838 = local read "Error code"() -> (w432:u16)
            n839 = property on="Reset" class="Bool"("Visible"=w436) -> ()  [unwired: 2 in, 2 out]
            n840 = property on="ERROR" class="Str"("Visible"=w436) -> ()  [unwired: 2 in, 2 out]
            n841 = Number To Decimal String(number=w432) -> (decimal integer string=w434:string)  [unwired: 1 in]
            n842 = case shown="0, Default" w432 {
              tunnel: ["Other error" ("ERROR") "Command buffer is full." ("ERROR") "The robot is not activated." ("ERROR") "The robot is not homed." ("ERROR") "Joint over limit." ("ERROR") "The robot is in error" ("ERROR") "Singularity detected." ("ERROR") "Activation failed." ("ERROR") "Homing failed" ("ERROR") "Pose out of reach." ("ERROR")] -> w430
              frame 0, Default {
                # "only show common error"
              }
              frame 1000 {
              }
              frame 1005 {
              }
              frame 1006 {
              }
              frame 1007 {
              }
              frame 1011 {
              }
              frame 1012 {
              }
              frame 1013 {
              }
              frame 1014 {
              }
              frame 1016 {
              }
            }
            n843 = Concatenate Strings("Error code: " ("ERROR"), w434, "\r\n", w430) -> (w433:string)
          }
          frame 3 {
            n844 = property on="ERROR" class="Str"("Visible"=TRUE) -> ()  [unwired: 2 in, 2 out]
          }
          frame 4 {
            n845 = property on="ERROR" class="Str"("Visible"=TRUE) -> ()  [unwired: 2 in, 2 out]
          }
        }
        n846 = property on="ERROR" class="Str"("Value"=w377) -> ()  [unwired: 2 in, 2 out]
        n847 = local read "Waiting"() -> (w383:bool)
        n848 = case shown="True" w383 {
          frame False {
          }
          frame True {
            n849 = shared-variable "Chan's target\\EtherCAT Master\\Device\\Robot Status-Activated"() -> (w420:bool)  [unwired: 1 in, 1 out]
            n850 = property on="Showbar" class="Bool (strict)"() -> ("Left"=w416:i32)  [unwired: 2 in, 2 out]
            n851 = Add(x=2, y=w416) -> (x+y=w415:i32)
            n852 = Not Equal?(x=w416, y=535) -> (x != y?=w422:bool)
            n853 = Select(t=w415, s=w422, f=103) -> (s? t:f=w412:i32)
            n854 = property on="Showbar" class="Bool (strict)"("Left"=w412) -> ()  [unwired: 2 in, 2 out]
            n855 = Select(t="Calibrating..." ("String"), s=w420, f="Activating..." ("String")) -> (s? t:f=w417:string)
            n856 = property on="progress" class="Bool"("Caption.Text"=w417) -> ()  [unwired: 2 in, 2 out]
          }
        }
        n857 = shared-variable "Chan's target\\EtherCAT Master\\Device\\Motion Status-Paused"() -> (w381:bool)  [unwired: 1 in, 1 out]
        n858 = call "Is Value Changed.vim"("value"=w381) -> ("changed or first call?"=w382:bool)
        n859 = case shown="True" w382 {
          tunnel: w381 -> [_ w411]
          frame False {
          }
          frame True {
            n860 = local write "Pause"(w411) -> ()
          }
        }
        n861 = Search Variable Container(7:w375, 11:refnum<k21> "ni.var.io:/" ("container refnum in")) -> (2:w361:refnum<k21>[])  [unwired: 4 in, 2 out]
        n862 = Index Array(array=w361, index=0) -> (element=w374:refnum<k21>)
        n863 = invoke class="IndComECAT Slave" method="neLVRefNum_Slave_GetState"(reference=w374) -> ("Slave State"=w373:u32)  [unwired: 5 in, 5 out]
        "Slave State" <- w373
        n864 = Not Equal?(x=w373, y=u32 8) -> (x != y?=w371:bool)
        n865 = case shown="True" w371 {
          selector: w371 -> [w408 w409]
          tunnel: [w408 w409] -> w370
          frame False {
          }
          frame True {
            n866 = One Button Dialog(message="Not in OP mode\n(Disconnected)") -> ()  [unwired: 1 in, 1 out]
          }
        }
        n867 = disable-structure shown="Enabled" {
          disable-tunnel: w370 -> [w405 w406]
          frame Disabled {
            n868 = Stop(stop? (T)=w405) -> ()
          }
          frame Enabled {
            n869 = local write "stop"(w406) -> ()
          }
        }
        n870 = case shown="True" "help" {
          frame False {
          }
          frame True {
            n871 = One Button Dialog(message="Shortcut\n--------------------------------------------------------------\nPages: F1~F6\nHoming: home\nStop : esc \nDevlopment  mode: Expand the window down and left\n--------------------------------------------------------------") -> ()  [unwired: 1 in, 1 out]
          }
        }
        n872 = First Call?() -> (First Call?: T/F=w359:bool)
        n873 = call "Is Value Changed.vim"("value"="Joints' Tor") -> ("changed or first call?"=w357:bool)
        n874 = Not(x=w359) -> (.not. x?=w358:bool)
        n875 = And(x=w358, y=w357) -> (x .and. y?=w356:bool)
        n876 = case shown="True" w356 {
          tunnel: "Joints' Tor" -> [_ w404]
          frame False {
          }
          frame True {
            n877 = property on="Torques" class="WFChart (strict)"("Visible"=w404) -> ()  [unwired: 2 in, 2 out]
          }
        }
        n878 = local read "stop"() -> (w367:bool)
      }
      n879 = node-c288(w147) -> ()  [unwired: 1 out]
      n880 = node-c288(w141) -> ()  [unwired: 1 out]
      n881 = node-c288(w149) -> ()  [unwired: 1 out]
      n882 = xnode "Read/Write Control"("FPGA VI Reference In"=w144, "CH1 DC"=fxp<+,32,0> 0.0 ("CH4 DC"), "ENA1"=w146, "STBY1"=w146) -> ("FPGA VI Reference Out"=w143:refnum<k20>)  [unwired: 1 in, 1 out]
      n883 = disable-structure shown="Disabled" {
        frame Disabled {
          n884 = while {
            stop <- w159 stop-if-true
            # "Repetitive exp - motion planning"
            n885 = local read "stop"() -> (w159:bool)
            n886 = feedback #25() -> (w157:dbl[][])  [unwired: 1 in]
            n887 = case shown="True" "plan" {
              selector: "plan" -> [_ w162]
              tunnel: [w160 w166] -> w158
              tunnel: w157 -> [w160 _]
              frame False {
              }
              frame True {
                n888 = call "Motion planning.vi"("Command"="Commands 2", "Root length"="Root length", "Section length"="Seccction length", "Times"="Times", "Set"=w162) -> ("Result"=w166:dbl[][])
              }
            }
            "Motions" <- w158
            n889 = feedback-in #25(w158) -> ()
          }
        }
        frame Enabled {
        }
      }
      n890 = xnode "Close FPGA VI Reference"("FPGA VI Reference In"=w143) -> ()  [unwired: 1 in, 1 out]
      n891 = node-c288(w153) -> ()  [unwired: 1 out]
      n892 = node-c288() -> (w140:T19)  [unwired: 4 in]
      n893 = timed-loop {
        timing: w140 -> [_]
        timing-out: [_] -> w139
        stop <- w275 stop-if-true
        w203 = dbl[] [0.0, 0.0, 0.0, 0.0, 0.0, 0.0]
        w225 = 3 ("index")
        w241 = dbl[] [0.0, 0.0, 0.0, 0.0, 0.0, 0.0]
        # "m to mm"
        # "m to mm"
        # "For command"
        # "For data record"
        # "Rt_S = Rt_6"
        # "Threshold should be considered in tool frame.\nHowever, we still need to  transform F/T from {t} to {6}"
        # "Admittance Control (Tustin)"
        n894 = node-c288() -> (w274:i64)  [unwired: 1 in]
        n895 = local read "External force_{t}"() -> (w231:T2)
        n896 = First Call?() -> (First Call?: T/F=w273:bool)
        n897 = case shown="True" w273 {
          tunnel: w274 -> [_ w281]
          frame False {
          }
          frame True {
            n898 = local read "scan engine"() -> (w279:u32)
            n899 = Square(x=i64 1000 ("value")) -> (x^2=w276:i64)
            n900 = Reciprocal(x=w276) -> (1/x=w278:dbl)
            n901 = Compound Arithmetic op=MULTIPLY(w281, w279, w278) -> (→"Sampling time (s)":dbl)
          }
        }
        n902 = Cluster To Array ("Cluster To Array 2")(cluster=w231) -> (array=w271:dbl[])
        n903 = Index Array(array="F_des", index=2) -> (element=w171:dbl)
        n904 = Add(x="F_des", y=w271) -> (x+y=w233:dbl[])
        n905 = global write "Fz_des.vi" "Fz_des"(w171) -> ()
        n906 = Absolute Value(x=w233) -> (abs(x)=w243:dbl[])
        n907 = Greater? ("Greater? 2")(x=w243, y="Threshold") -> (0:w238:bool[])
        n908 = Or Array Elements(Boolean array=w238) -> (logical OR=→"Moving?":bool)
        n909 = Boolean To (0,1)(Boolean=w238) -> (0, 1=w244:i16[])
        n910 = To Double Precision Float(number=w244) -> (double precision float=w245:dbl[])
        n911 = Multiply ("Multiply 2")(x=w233, y=w245) -> (x*y=w180:dbl[])
        n912 = local read "Rt_S"() -> (w222:dbl[][])
        n913 = Transpose 2D Array(2D array=w222) -> (transposed array=w226:dbl[][])
        n914 = Array Subset(array=w180, index=w225, length=w225) -> (w227:dbl[])
        n915 = Array Subset(array=w180, index=0, length=3) -> (w228:dbl[])
        n916 = call-poly <vilib>:"A x B.vi"("Vector"=w227, "A"=w226) -> ("A x Vector"=w223:dbl[])  [unwired: 1 out]
        n917 = call-poly <vilib>:"A x B.vi"("Vector"=w228, "A"=w226) -> ("A x Vector"=w224:dbl[])  [unwired: 1 out]
        n918 = Build Array (concatenate)(w224, w223) -> (w181:dbl[])
        n919 = local read "time constant"() -> (w186:dbl)
        n920 = local read "Drag"() -> (w202:bool)
        n921 = local read "Drag"() -> (w242:bool)
        n922 = local read "Sampling time (s)"() -> (w200:dbl)
        n923 = local read "Bi"() -> (w185:dbl[])
        n924 = local read "Sampling time (s)"() -> (w206:dbl)
        n925 = local read "Sampling time (s)"() -> (w248:dbl)
        n926 = Select(t=w180, s=w202, f=w203) -> (s? t:f=w221:dbl[])
        n927 = Select(t=w181, s=w242, f=w241) -> (s? t:f=w232:dbl[])
        n928 = Multiply(x=w185, y=w186) -> (x*y=w204:dbl[])
        n929 = Multiply(x="Bi", y="time constant") -> (x*y=w237:dbl[])
        "Mi" <- w237
        n930 = global write "Sensor_Force.vi" "Sensor_{t}_threshold"(w221) -> ()
        n931 = feedback #26(w203) -> (w189:dbl[])
        n932 = feedback-in #26(w221) -> ()
        n933 = feedback-in #27(w232) -> ()
        n934 = feedback #27(w241) -> (w270:dbl[])
        n935 = feedback #28(dbl[] [0.0, 0.0, 0.0, 0.0, 0.0, 0.0]) -> (w211:dbl[])
        n936 = feedback-in #28(w221) -> ()
        n937 = Add(x=w221, y=w189) -> (x+y=w192:dbl[])
        n938 = Add(x=w232, y=w270) -> (x+y=w267:dbl[])
        n939 = Multiply(x=w204, y=2.0 ("Numeric Control")) -> (x*y=w191:dbl[])
        n940 = local read "k"() -> (w183:dbl)
        n941 = Add(x=w221, y=w211) -> (x+y=w210:dbl[])
        n942 = Multiply(x=w200, y=w185) -> (x*y=w190:dbl[])
        n943 = Multiply(x=w237, y=2.0 ("Numeric Control")) -> (x*y=w268:dbl[])
        n944 = Multiply(x=w248, y="Bi") -> (x*y=w269:dbl[])
        n945 = Compound Arithmetic op=MULTIPLY(w183, w192, w200) -> (w195:dbl[])
        n946 = Compound Arithmetic op=MULTIPLY(w210, w206, 0.5 ("Numeric Control")) -> (w208:dbl[])
        n947 = Compound Arithmetic op=MULTIPLY("k", w267, w248) -> (w264:dbl[])
        n948 = Subtract(x=w190, y=w191) -> (x-y=w194:dbl[])
        n949 = Add(x=w190, y=w191) -> (x+y=w188:dbl[])
        n950 = Subtract(x=w269, y=w268) -> (x-y=w265:dbl[])
        n951 = Add(x=w269, y=w268) -> (x+y=w272:dbl[])
        n952 = local read "Joints(degree)"() -> (w258:T3)
        n953 = feedback #29(dbl[] [0.0, 0.0, 0.0, 0.0, 0.0, 0.0]) -> (w207:dbl[])
        n954 = Add(x=w208, y=w207) -> (x+y=w187:dbl[])
        "Impulse(J)" <- w187
        n955 = feedback-in #29(w187) -> ()
        n956 = feedback #30(dbl[] [0.0, 0.0, 0.0, 0.0, 0.0, 0.0]) -> (w193:dbl[])
        n957 = Multiply(x=w194, y=w193) -> (x*y=w196:dbl[])
        n958 = Reciprocal(x=w188) -> (1/x=w198:dbl[])
        n959 = Subtract(x=w195, y=w196) -> (x-y=w197:dbl[])
        n960 = feedback #31(dbl[] [0.0, 0.0, 0.0, 0.0, 0.0, 0.0]) -> (w266:dbl[])
        n961 = Multiply(x=w265, y=w266) -> (x*y=w263:dbl[])
        n962 = Reciprocal(x=w272) -> (1/x=w261:dbl[])
        n963 = Subtract(x=w264, y=w263) -> (x-y=w262:dbl[])
        n964 = Multiply(x=w197, y=w198) -> (x*y=w175:dbl[])
        n965 = feedback-in #30(w175) -> ()
        n966 = global write "Sensor_Impluse.vi" "Impulse(J)"(w187) -> ()
        n967 = Multiply(x=w262, y=w261) -> (x*y=w178:dbl[])
        n968 = feedback-in #31(w178) -> ()
        n969 = Cluster To Array(cluster=w258) -> (array=w169:sgl[])
        n970 = call "Meca_Jocobian.vi"("Joints"=w169) -> ("J-"=w259:dbl[][])  [unwired: 3 out]
        n971 = local read "Sampling time (s)"() -> (w217:dbl)
        n972 = Multiply(x=w178, y=1000.0) -> (x*y=w177:dbl[])
        n973 = Multiply(x=w175, y=1000.0) -> (x*y=w173:dbl[])
        "Vel_{t} (mm/s)" <- w173
        n974 = local read "Sampling time (s)"() -> (w249:dbl)
        n975 = call-poly <vilib>:"A x B.vi"("Vector"=w177, "A"=w259) -> ("A x Vector"=w184:dbl[])  [unwired: 1 out]
        "w" <- w184
        n976 = feedback #32(dbl[] [0.0, 0.0, 0.0, 0.0, 0.0, 0.0]) -> (w212:dbl[])
        n977 = feedback-in #32(w173) -> ()
        n978 = global write "Command_Velocity.vi" "Command_Velocity"(w173) -> ()
        n979 = Add(x=w173, y=w212) -> (x+y=w213:dbl[])
        n980 = feedback #33(dbl[] [0.0, 0.0, 0.0, 0.0, 0.0, 0.0]) -> (w257:dbl[])
        n981 = feedback-in #33(w184) -> ()
        n982 = Add(x=w184, y=w257) -> (x+y=w255:dbl[])
        n983 = Compound Arithmetic op=MULTIPLY(w213, w217, 0.5 ("Numeric Control")) -> (w215:dbl[])
        n984 = Compound Arithmetic op=MULTIPLY(w255, w249, 0.5 ("Numeric Control")) -> (w253:dbl[])
        n985 = feedback #34(dbl[] [0.0, 0.0, 0.0, 0.0, 0.0, 0.0]) -> (w216:dbl[])
        n986 = Add(x=w215, y=w216) -> (x+y=w179:dbl[])
        "Pos_{t} (mm)" <- w179
        n987 = feedback-in #34(w179) -> ()
        n988 = feedback #35(dbl[] [0.0, 0.0, 0.0, 0.0, 0.0, 0.0]) -> (w252:dbl[])
        n989 = Add(x=w253, y=w252) -> (x+y=w168:dbl[])
        "£c" <- w168
        n990 = feedback-in #35(w168) -> ()
        n991 = global write "Command_Position.vi" "Command_Position"(w179) -> ()
        n992 = feedback #36(dbl[] [0.0, 0.0, 0.0, 0.0, 0.0, 0.0]) -> (w250:dbl[])
        n993 = feedback-in #36(w168) -> ()
        n994 = Subtract(x=w168, y=w250) -> (x-y=w251:dbl[])
        n995 = local read "stop"() -> (w275:bool)
        n996 = Add(x=w169, y=w251) -> (x+y=→"Adm_joints":dbl[])
        n997 = node-c288() -> ()  [unwired: 1 in, 1 out]
      }
      n998 = node-c288(w151) -> ()  [unwired: 1 out]
      n999 = while {
        stop <- w465 stop-if-true
        # "Torque plot"
        n1000 = local read "Torque Ratio"() -> (w463:T3)
        n1001 = property on="Torques" class="WFChart (strict)"("Val(Sgnl)"=w463) -> ()  [unwired: 2 in, 2 out]
        n1002 = local read "stop"() -> (w465:bool)
        n1003 = Wait Until Next ms Multiple(millisecond multiple=u32 1) -> ()  [unwired: 1 out]
      }
      n1004 = node-c288(w139) -> ()  [unwired: 1 out]
    }
    frame #2 {
      # "Reset"
      n1005 = node-c288() -> (w1200:T19)  [unwired: 4 in]
      n1006 = timed-loop {
        timing: w1200 -> [_]
        timing-out: [_] -> w1199
        i -> [w1202]
        stop <- w1203 stop-if-true
        # "Clear commands"
        n1007 = node-c288() -> ()  [unwired: 1 in, 1 out]
        n1008 = case shown="5, 6" w1202 {
          frame 0..2, Default {
            n1009 = shared-variable "Chan's target\\EtherCAT Master\\Device\\Motion Control-Clear Move"(TRUE ("Motion Control-Clear Move")) -> ()  [unwired: 1 in, 1 out]
          }
          frame 3, 4 {
            n1010 = shared-variable "Chan's target\\EtherCAT Master\\Device\\Motion Control-Pause"(FALSE ("Motion Control-Pause")) -> ()  [unwired: 1 in, 1 out]
          }
          frame 5, 6 {
            n1011 = shared-variable "Chan's target\\EtherCAT Master\\Device\\Motion Control-Clear Move"(FALSE ("Motion Control-Clear Move")) -> ()  [unwired: 1 in, 1 out]
          }
        }
        n1012 = Equal?(x=w1202, y=7) -> (x = y?=w1203:bool)
        n1013 = node-c288() -> ()  [unwired: 1 in, 1 out]
      }
      n1014 = node-c288(w1199) -> ()  [unwired: 1 out]
    }
  }
